vi "Configure_Run.vi"(8 "error in":errorcluster, 9 "Base Station":T1="BS1", 10 "Band":enum32{"GSM", "eNodeB", "gNodeB"}(ring)=enum."eNodeB", 11 "Input":T2={"Ref_Cluster"={"UE1"=refnum, "UE2"=refnum, "UE3"=refnum, "SelectNetwork1"=refnum, "SelectNetwork3"=refnum, "SelectNetwork2"=refnum, "Trace_Table1"=refnum, "UE - 1"=refnum, "UE - 2"=refnum, "UE - 3"=refnum, "UE - 4"=refnum, "Network-3"=refnum, "Status"=refnum, "Trace_Table2"=refnum, "UE4"=refnum, "Start"=refnum, "Reset"=refnum, "IP simulation"=refnum, "Network-1"=refnum, "Time Stamp"=refnum, "Network-2"=refnum, "IMS"=refnum, "GSM-Data"=refnum, "Configurations"=refnum, "Band"=refnum, "Sim Configurations"=refnum, "ECall"=refnum, "WWW"=refnum, "Cancel Configurations"=refnum, "GSM-PHY"=refnum, "GSM-CELL"=refnum, "GSM-GPRS"=refnum, "LTE-CELL"=refnum, "LTE-PHY"=refnum, "LTE-RRC"=refnum, "LTE-SDR"=refnum, "NR-RRC"=refnum, "NR-SDR"=refnum, "NR-PHY"=refnum, "NR-CELL"=refnum, "GSM-SDR"=refnum, "gNodeB-Data"=refnum, "eNodeB-Data"=refnum, "Select BS"=refnum, "Download"=refnum, "Upload"=refnum}, "Time Stamp"=timestamp(0 s since 1904-01-01), "Network-3"={"NW3-Thr-Down"=0.0, "NW3-Thr-Up"=0.0, "NW3-Fre-Down"=0.0, "NW3-Fre-Up"=0.0, "NW3-PwL-Down"=0.0, "NW3-PwL-Up"=0.0}, "Network-2"={"NW2-Thr-Down"=0.0, "NW2-Thr-Up"=0.0, "NW2-Fre-Down"=0.0, "NW2-Fre-Up"=0.0, "NW2-PwL-Down"=0.0, "NW2-PwL-Up"=0.0}, "Network-1"={"NW1-Thr-Down"=0.0, "NW1-Thr-Up"=0.0, "NW1-Fre-Down"=0.0, "NW1-Fre-Up"=0.0, "NW1-PwL-Down"=0.0, "NW1-PwL-Up"=0.0}, "UE - 4"={"UE4-Idle"=FALSE, "UE4-Origination"=FALSE, "UE4-Registration"=FALSE, "UE4-Pdu Connection"=FALSE, "UE4-Termination"=FALSE, "UE4-Detach"=FALSE}, "UE - 2"={"UE2-Idle"=FALSE, "UE2-Origination"=FALSE, "UE2-Registration"=FALSE, "UE2-Pdu Connection"=FALSE, "UE2-Termination"=FALSE, "UE2-Detach"=FALSE}, "UE - 1"={"UE1-Idle"=FALSE, "UE1-Origination"=FALSE, "UE1-Registration"=FALSE, "UE1-Pdu Connection"=FALSE, "UE1-Termination"=FALSE, "UE1-Detach"=FALSE}, "UE - 3"={"UE3-Idle"=FALSE, "UE3-Origination"=FALSE, "UE3-Registration"=FALSE, "UE3-Pdu Connection"=FALSE, "UE3-Termination"=FALSE, "UE3-Detach"=FALSE}, "IP simulation"=FALSE, "Start"=FALSE, "Reset"=FALSE, "Download"=FALSE, "Upload"=FALSE, "UE4"=FALSE, "UE3"=FALSE, "UE2"=FALSE, "UE1"=FALSE, "Trace_Table1"=0, "Status"="", "Trace_Table2"=0, "SelectNetwork1"={"Nw1-check"=FALSE, "NW-Combo"="GSM"}, "SelectNetwork2"={"Nw1-check"=FALSE, "NW-Combo"="GSM"}, "SelectNetwork3"={"Nw1-check"=FALSE, "NW-Combo"="GSM"}, "IMS"=FALSE, "WWW"=FALSE, "Sim Configuration"=FALSE, "Ecall"=FALSE, "Configurations"=enum."Configurations", "Band"=enum."GSM", "GSM-Data"=enum."SDR", "eNodeB-Data"=enum."RRC", "gNodeB-Data"=enum."SDR", "Cancel Configurations"=FALSE, "IP_UI"={"Add"=FALSE, "Close"=FALSE, "IP_UI"=[]}, "IMS_DATA"=[], "ECall DATA"=[], "Technology"="", "Sim Cluster in"={"Session_array"=[{"Add Bearer"=FALSE, "APN Name\n"="as", "AMBR Uplink(Gbps)\n"="as", "AMBR Downlink(Gbps)\n"="11111111111111111111111111111111", "Session name"="8baf473f2f8fd09487cccbd7097c6862", "Bearer_Array"=[], "Delete Session"=FALSE}], "SIM_U_Config"={"Add"=FALSE, "Close"=TRUE, "SIM_UI"=[], "Save"=FALSE}}, "Select BS"="", "Select Network 1"={"Network 1-2G"={"GSM-SDR"={"DL Reference Power"=-13, "Serail Name"="", "UL Reference Power"=-13, "Radio Device"="0"}, "GSM-GPRS"={"Priority Access THR"="6", "Acess Burst Type"="0", "Nack Countdown"="8", "BCCH/PDCH Measurement"="0", "Routing Area Code(RAC)"=128, "Network Control Order"="0", "t3168"="3", "t3192"="2", "Alpha"="10"}, "GSM-PHY"={"RACH Maximum Retransmission"="3", "RACH Transmission Slots"="1", "RACH Call Reestablishment"="1", "RACH Access Control Class"="1", "Block for Access Grant"="0", "Multiframe for Paging"="0", "Power Control Indicator"="0", "Radio Link Timeout"="850", "Cell Reselect Hysterisis"="0", "Attach/Detach Allowed"="0", "CCCH Combinations"="0", "t3212"=0, "DTX Indicator"="1", "Power Control Level"=0, "Minimum Received Signal Level"=0, "Half Rate Support"="0", "Add Reselect"="1"}, "GSM-CELL"={"SMS Enabled"="0", "Eutra Operating Bands"="3", "Power Offset Indicator"="", "Early Classmark Sending Control"="1", "Location Area Code"=0, "CALL Enabled"="1", "Loop Back Enabled"="0", "GPRS Enabled"="1", "SI Type 2 ter Indicator"="0", "ARFCN"=1, "Frequency Format ID"=1, "Mobile Country Code"=1, "Mobile Network Code"=1, "Cell Barred Access"="ONESIXTH", "Downlink Frequency"=-13, "Uplink Frequency"=1842}}, "Network 1-4G"={"LTE-SDR"={"Radio Device"="0", "DL Reference Power"=-13, "Serail Name"="", "UL Reference Power"=-13, "DL Antennas"="1", "UL Antennas"="1"}, "LTE-PHY"={"PBCH Repetition"="0", "PUCCH Delta Shift"="0", "PUCCH CQI Number of RB"="2", "PHICH Resource"="0", "SRS Enable"="0", "PCCH Paging Cycle"="1", "BCCH Modification Coefficient"="10", "PUSCH Alpha"="48", "PUSCH DMRS Enable"="4", "PHICH Duration"="10", "PUCCH HARQ Max Transmission"=-27, "PCCH Narrowband Count"="-108", "PUSCH Power Offset"=0, "PUCCH Power Offset"=0, "PDSCH Power Boost"="0", "PUCCH An Occassions"="1", "PUUCH CS Antenna Ports"="10", "PRACH Response Window Size"="MaxEye", "PRACH Contention Resolution Timer"="TM1", "PRACH Ramping Step Size"="2", "PDSCH Reference Power"=-27, "PRACH Root Sequence Index"=80, "PRACH Maximum Transmissions"="0", "PRACH Initial Received Target Power"="4", "PRACH Configuration Index"=98}, "LTE-CELL"={"Duplex Mode"="10", "Measurement Report"="1", "Eutra Operating Bands"="139", "Carrier Bandwidth"="10", "Physical Cell ID"=0, "Network Name"="one", "DL Frequency"=4, "UL Frequency"=25, "Transmission Mode"="TM1", "MNC Length"="77", "IMS Enabled"="1", "Tracking Area Code"=1, "Mobile Network Code"=1, "Mobile Country Code"=1}, "LTE-RRC"={"RLC Maximum Retransmision Threshold"="1", "RLC Timer Poll Retransmit"=0, "RLC Timer Reordering"=0, "RLC Timer Status Prohibit"=-96, "RLC Poll PDU"=13, "RLC Poll Byte"=1}}, "Network 1-5G"={"NR-SDR"={"DL Reference Power"=0, "Serail Name"="1", "UL Reference Power"=-13, "DL Antennas"="0", "UL Antennas"="0", "Radio Device"="1"}, "NR-PHY"={"PDSCH Reference Power"=-27, "SSB RSRP Threshold"=-109, "PRACH Contention Resolution Timer"=7, "Preamble Per SSB"=14, "Preamble Per SSB Format"=4, "UE Power Level Grant"=-90, "RA Response Window"="1", "Power Ramp Step Size"="2", "Preamble Root Sequence Index"="139", "Preamble Transmission Count"="10", "Preamble Received Power"=-96, "Zero Correlation Zone Configuration"=13, "Msg Frequency Division Multiplexing"="one", "PRACH Configuration Index"=98, "Preamble Timing Offset"=1, "Preamble Format"=0, "Resource Restriction Type"="0"}, "NR-CELL"={"Tracking Area Code"=1, "Mobile Country Code"=1, "Mobile Network Code"=1, "Operating Bands"="77", "Physical Cell ID"=0, "DL Offset to Carrier"=0, "Subcarrier Spacing"="1", "UL Offset to Carrier 2"=0, "Carrier Bandwidth"="10", "Transmission Mode"="TM1", "CSI-RS"="1", "SRS"="1", "Measurement Report"="1"}, "NR-RRC"={"Ciphering Algorithms for SRB"="0", "Integrity Algorithms for SRB"="0", "Ciphering Algorithms for DRB"="1", "Integrity Algorithms for DRB"="1"}}, "Technology-1"=""}, "Select Network 2"={"Network 2-2G"={"GSM-SDR"={"DL Reference Power"=-13, "Serail Name"="", "UL Reference Power"=-13, "Radio Device"="0"}, "GSM-GPRS"={"Priority Access THR"="6", "Acess Burst Type"="0", "Nack Countdown"="8", "BCCH/PDCH Measurement"="0", "Routing Area Code(RAC)"=128, "Network Control Order"="0", "t3168"="3", "t3192"="2", "Alpha"="10"}, "GSM-PHY"={"RACH Maximum Retransmission"="1", "RACH Transmission Slots"="14", "RACH Call Reestablishment"="1", "RACH Access Control Class"="0", "Block for Access Grant"="2", "Multiframe for Paging"="0", "Power Control Indicator"="0", "Radio Link Timeout"="15", "Cell Reselect Hysterisis"="3", "Attach/Detach Allowed"="1", "CCCH Combinations"="1", "t3212"=0, "DTX Indicator"="1", "Power Control Level"=0, "Minimum Received Signal Level"=0, "Half Rate Support"="0", "Add Reselect"="0"}, "GSM-CELL"={"SMS Enabled"="0", "Eutra Operating Bands"="850", "Power Offset Indicator"="0", "Early Classmark Sending Control"="0", "Location Area Code"=1, "CALL Enabled"="0", "Loop Back Enabled"="1", "GPRS Enabled"="0", "SI Type 2 ter Indicator"="1", "ARFCN"=0, "Frequency Format ID"=71, "Mobile Country Code"=1, "Mobile Network Code"=1, "Cell Barred Access"="0", "Downlink Frequency"=0, "Uplink Frequency"=900200000}}, "Network 2-4G"={"LTE-SDR"={"Radio Device"="0", "DL Reference Power"=-13, "Serail Name"="", "UL Reference Power"=-13, "DL Antennas"="1", "UL Antennas"="1"}, "LTE-PHY"={"PBCH Repetition"="0", "PUCCH Delta Shift"="1", "PUCCH CQI Number of RB"="0", "PHICH Resource"="ONESIXTH", "SRS Enable"="0", "PCCH Paging Cycle"="256", "BCCH Modification Coefficient"="2", "PUSCH Alpha"="1", "PUSCH DMRS Enable"="0", "PHICH Duration"="0", "PUCCH HARQ Max Transmission"=4, "PCCH Narrowband Count"="2", "PUSCH Power Offset"=-96, "PUCCH Power Offset"=-96, "PDSCH Power Boost"="0", "PUCCH An Occassions"="0", "PUUCH CS Antenna Ports"="1", "PRACH Response Window Size"="10", "PRACH Contention Resolution Timer"="48", "PRACH Ramping Step Size"="4", "PDSCH Reference Power"=-27, "PRACH Root Sequence Index"=0, "PRACH Maximum Transmissions"="10", "PRACH Initial Received Target Power"="-108", "PRACH Configuration Index"=0}, "LTE-CELL"={"Duplex Mode"="0", "Measurement Report"="1", "Eutra Operating Bands"="3", "Carrier Bandwidth"="10", "Physical Cell ID"=0, "Network Name"="MaxEye", "DL Frequency"=1842, "UL Frequency"=1747, "Transmission Mode"="TM1", "MNC Length"="2", "IMS Enabled"="0", "Tracking Area Code"=1, "Mobile Network Code"=1, "Mobile Country Code"=1}, "LTE-RRC"={"RLC Maximum Retransmision Threshold"="4", "RLC Timer Poll Retransmit"=80, "RLC Timer Reordering"=35, "RLC Timer Status Prohibit"=0, "RLC Poll PDU"=4, "RLC Poll Byte"=25}}, "Network 2-5G"={"NR-SDR"={"DL Reference Power"=-13, "Serail Name"="", "UL Reference Power"=-13, "DL Antennas"="1", "UL Antennas"="1", "Radio Device"="0"}, "NR-PHY"={"PDSCH Reference Power"=-27, "SSB RSRP Threshold"=-109, "PRACH Contention Resolution Timer"=7, "Preamble Per SSB"=14, "Preamble Per SSB Format"=4, "UE Power Level Grant"=-90, "RA Response Window"="10", "Power Ramp Step Size"="2", "Preamble Root Sequence Index"="139", "Preamble Transmission Count"="10", "Preamble Received Power"=-96, "Zero Correlation Zone Configuration"=13, "Msg Frequency Division Multiplexing"="one", "PRACH Configuration Index"=98, "Preamble Timing Offset"=1, "Preamble Format"=0, "Resource Restriction Type"="0"}, "NR-CELL"={"Tracking Area Code"=1, "Mobile Country Code"=1, "Mobile Network Code"=1, "Operating Bands"="77", "Physical Cell ID"=0, "DL Offset to Carrier"=0, "Subcarrier Spacing"="1", "UL Offset to Carrier 2"=0, "Carrier Bandwidth"="10", "Transmission Mode"="TM1", "CSI-RS"="1", "SRS"="1", "Measurement Report"="1"}, "NR-RRC"={"Ciphering Algorithms for SRB"="0", "Integrity Algorithms for SRB"="0", "Ciphering Algorithms for DRB"="1", "Integrity Algorithms for DRB"="1"}}, "Technology-2"=""}, "Select Network 3"={"Network 3-2G"={"GSM-SDR"={"DL Reference Power"=-13, "Serail Name"="", "UL Reference Power"=-13, "Radio Device"="0"}, "GSM-GPRS"={"Priority Access THR"="6", "Acess Burst Type"="0", "Nack Countdown"="8", "BCCH/PDCH Measurement"="0", "Routing Area Code(RAC)"=128, "Network Control Order"="0", "t3168"="3", "t3192"="2", "Alpha"="10"}, "GSM-PHY"={"RACH Maximum Retransmission"="1", "RACH Transmission Slots"="14", "RACH Call Reestablishment"="1", "RACH Access Control Class"="0", "Block for Access Grant"="2", "Multiframe for Paging"="0", "Power Control Indicator"="0", "Radio Link Timeout"="15", "Cell Reselect Hysterisis"="3", "Attach/Detach Allowed"="1", "CCCH Combinations"="1", "t3212"=0, "DTX Indicator"="1", "Power Control Level"=0, "Minimum Received Signal Level"=0, "Half Rate Support"="0", "Add Reselect"="0"}, "GSM-CELL"={"SMS Enabled"="0", "Eutra Operating Bands"="850", "Power Offset Indicator"="0", "Early Classmark Sending Control"="0", "Location Area Code"=1, "CALL Enabled"="0", "Loop Back Enabled"="1", "GPRS Enabled"="0", "SI Type 2 ter Indicator"="1", "ARFCN"=0, "Frequency Format ID"=71, "Mobile Country Code"=1, "Mobile Network Code"=1, "Cell Barred Access"="0", "Downlink Frequency"=0, "Uplink Frequency"=900200000}}, "Network 3-4G"={"LTE-SDR"={"Radio Device"="0", "DL Reference Power"=-13, "Serail Name"="", "UL Reference Power"=-13, "DL Antennas"="1", "UL Antennas"="1"}, "LTE-PHY"={"PBCH Repetition"="0", "PUCCH Delta Shift"="1", "PUCCH CQI Number of RB"="0", "PHICH Resource"="ONESIXTH", "SRS Enable"="0", "PCCH Paging Cycle"="256", "BCCH Modification Coefficient"="2", "PUSCH Alpha"="1", "PUSCH DMRS Enable"="0", "PHICH Duration"="0", "PUCCH HARQ Max Transmission"=4, "PCCH Narrowband Count"="2", "PUSCH Power Offset"=-96, "PUCCH Power Offset"=-96, "PDSCH Power Boost"="0", "PUCCH An Occassions"="0", "PUUCH CS Antenna Ports"="1", "PRACH Response Window Size"="10", "PRACH Contention Resolution Timer"="48", "PRACH Ramping Step Size"="4", "PDSCH Reference Power"=-27, "PRACH Root Sequence Index"=0, "PRACH Maximum Transmissions"="10", "PRACH Initial Received Target Power"="-108", "PRACH Configuration Index"=0}, "LTE-CELL"={"Duplex Mode"="0", "Measurement Report"="1", "Eutra Operating Bands"="3", "Carrier Bandwidth"="10", "Physical Cell ID"=0, "Network Name"="MaxEye", "DL Frequency"=1842, "UL Frequency"=1747, "Transmission Mode"="TM1", "MNC Length"="2", "IMS Enabled"="0", "Tracking Area Code"=1, "Mobile Network Code"=1, "Mobile Country Code"=1}, "LTE-RRC"={"RLC Maximum Retransmision Threshold"="4", "RLC Timer Poll Retransmit"=80, "RLC Timer Reordering"=35, "RLC Timer Status Prohibit"=0, "RLC Poll PDU"=4, "RLC Poll Byte"=25}}, "Network 3-5G"={"NR-SDR"={"DL Reference Power"=-13, "Serail Name"="", "UL Reference Power"=-13, "DL Antennas"="1", "UL Antennas"="1", "Radio Device"="0"}, "NR-PHY"={"PDSCH Reference Power"=-27, "SSB RSRP Threshold"=-109, "PRACH Contention Resolution Timer"=7, "Preamble Per SSB"=14, "Preamble Per SSB Format"=4, "UE Power Level Grant"=-90, "RA Response Window"="10", "Power Ramp Step Size"="2", "Preamble Root Sequence Index"="139", "Preamble Transmission Count"="10", "Preamble Received Power"=-96, "Zero Correlation Zone Configuration"=13, "Msg Frequency Division Multiplexing"="one", "PRACH Configuration Index"=98, "Preamble Timing Offset"=1, "Preamble Format"=0, "Resource Restriction Type"="0"}, "NR-CELL"={"Tracking Area Code"=1, "Mobile Country Code"=1, "Mobile Network Code"=1, "Operating Bands"="77", "Physical Cell ID"=0, "DL Offset to Carrier"=0, "Subcarrier Spacing"="1", "UL Offset to Carrier 2"=0, "Carrier Bandwidth"="10", "Transmission Mode"="TM1", "CSI-RS"="1", "SRS"="1", "Measurement Report"="1"}, "NR-RRC"={"Ciphering Algorithms for SRB"="0", "Integrity Algorithms for SRB"="0", "Ciphering Algorithms for DRB"="1", "Integrity Algorithms for DRB"="1"}}, "Technology-3"=""}, "Current Technology"="", "Current Network"=""} {"Time Stamp" format="%<%H:%M:%S>T"}) -> (0 "error out":errorcluster)   [LabVIEW 2021]
uses:
  Controls/ATE_BSE_Controls_ref.ctl
  Controls/ATE_BSE_ref_type_Def.ctl
  IP Simulation/Controls/IP_Cellular Tech Type def.ctl
  IP Simulation/Controls/IP_Network_Type def.ctl
  IP Simulation/Controls/IP_Type-Tydedef.ctl
  Save File/Sim_Confi.ctl
  APIs/Controls/Base_Station_Emulator.ctl
  APIs/Controls/Cellular_Technology.ctl
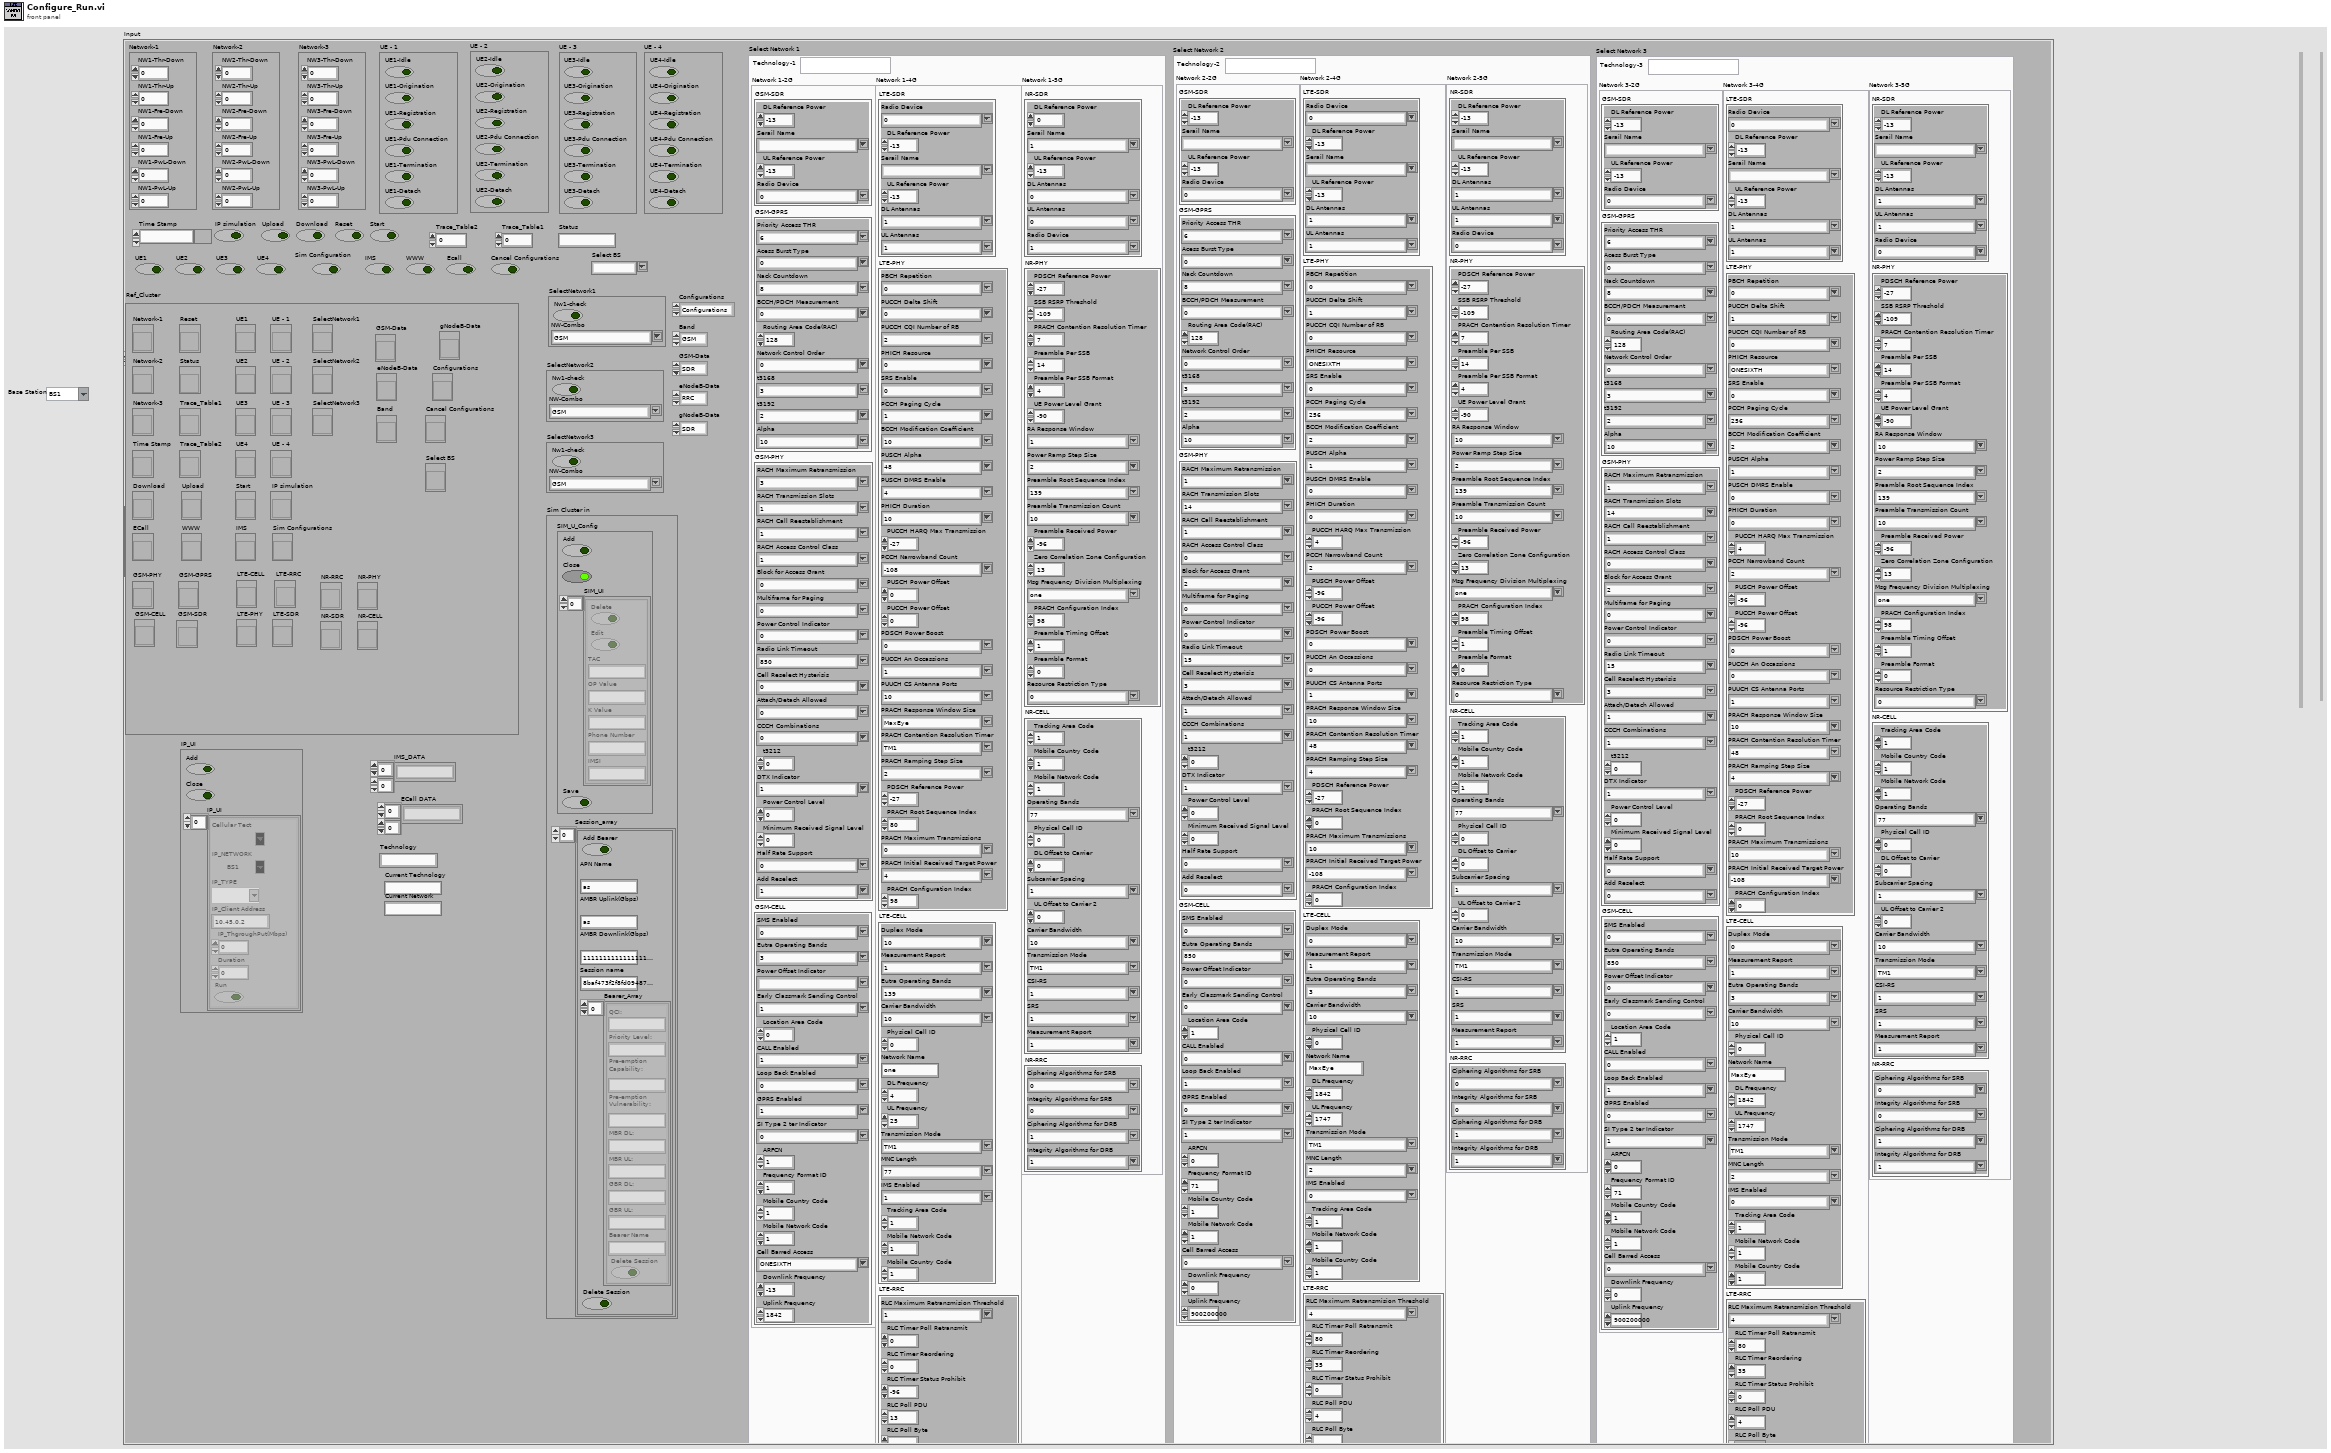
[diagram p1: front panel]
types:
  T1 = typedef "Base_Station_Emulator.ctl" = string
  T2 = typedef "ATE_BSE_Controls_ref.ctl" = cluster{"Ref_Cluster":T3, "Time Stamp":timestamp, "Network-3":cluster{"NW3-Thr-Down":dbl, "NW3-Thr-Up":dbl, "NW3-Fre-Down":dbl, "NW3-Fre-Up":dbl, "NW3-PwL-Down":dbl, "NW3-PwL-Up":dbl}, "Network-2":cluster{"NW2-Thr-Down":dbl, "NW2-Thr-Up":dbl, "NW2-Fre-Down":dbl, "NW2-Fre-Up":dbl, "NW2-PwL-Down":dbl, "NW2-PwL-Up":dbl}, "Network-1":cluster{"NW1-Thr-Down":dbl, "NW1-Thr-Up":dbl, "NW1-Fre-Down":dbl, "NW1-Fre-Up":dbl, "NW1-PwL-Down":dbl, "NW1-PwL-Up":dbl}, "UE - 4":cluster{"UE4-Idle":bool, "UE4-Origination":bool, "UE4-Registration":bool, "UE4-Pdu Connection":bool, "UE4-Termination":bool, "UE4-Detach":bool}, "UE - 2":cluster{"UE2-Idle":bool, "UE2-Origination":bool, "UE2-Registration":bool, "UE2-Pdu Connection":bool, "UE2-Termination":bool, "UE2-Detach":bool}, "UE - 1":cluster{"UE1-Idle":bool, "UE1-Origination":bool, "UE1-Registration":bool, "UE1-Pdu Connection":bool, "UE1-Termination":bool, "UE1-Detach":bool}, "UE - 3":cluster{"UE3-Idle":bool, "UE3-Origination":bool, "UE3-Registration":bool, "UE3-Pdu Connection":bool, "UE3-Termination":bool, "UE3-Detach":bool}, "IP simulation":bool, "Start":bool, "Reset":bool, "Download":bool, "Upload":bool, "UE4":bool, "UE3":bool, "UE2":bool, "UE1":bool, "Trace_Table1":i32, "Status":string, "Trace_Table2":i32, "SelectNetwork1":cluster{"Nw1-check":bool, "NW-Combo":string}, "SelectNetwork2":cluster{"Nw1-check":bool, "NW-Combo":string}, "SelectNetwork3":cluster{"Nw1-check":bool, "NW-Combo":string}, "IMS":bool, "WWW":bool, "Sim Configuration":bool, "Ecall":bool, "Configurations":enum32{"Configurations", "Main"}, "Band":enum32{"GSM", "gNodeB", "eNodeB"}, "GSM-Data":enum32{"SDR", "CELL", "PHY", "GPRS"}, "eNodeB-Data":enum32{"SDR", "CELL", "PHY", "RRC"}, "gNodeB-Data":enum32{"SDR", "CELL", "PHY", "RRC"}, "Cancel Configurations":bool, "IP_UI":cluster{"Add":bool, "Close":bool, "IP_UI":cluster{"Cellular Tect":T4, "IP_NETWORK":T5, "IP_TYPE":T6, "IP_Client Address":string, "IP_ThgroughPut(Mbps)":i32, "Duration":i32, "Run":bool}[]}, "IMS_DATA":string[][], "ECall DATA":string[][], "Technology":string, "Sim Cluster in":T7, "Select BS":string, "Select Network 1":cluster{"Network 1-2G":cluster{"GSM-SDR":cluster{"DL Reference Power":i32, "Serail Name":string, "UL Reference Power":i32, "Radio Device":string}, "GSM-GPRS":cluster{"Priority Access THR":string, "Acess Burst Type":string, "Nack Countdown":string, "BCCH/PDCH Measurement":string, "Routing Area Code(RAC)":i32, "Network Control Order":string, "t3168":string, "t3192":string, "Alpha":string}, "GSM-PHY":cluster{"RACH Maximum Retransmission":string, "RACH Transmission Slots":string, "RACH Call Reestablishment":string, "RACH Access Control Class":string, "Block for Access Grant":string, "Multiframe for Paging":string, "Power Control Indicator":string, "Radio Link Timeout":string, "Cell Reselect Hysterisis":string, "Attach/Detach Allowed":string, "CCCH Combinations":string, "t3212":i64, "DTX Indicator":string, "Power Control Level":i64, "Minimum Received Signal Level":i64, "Half Rate Support":string, "Add Reselect":string}, "GSM-CELL":cluster{"SMS Enabled":string, "Eutra Operating Bands":string, "Power Offset Indicator":string, "Early Classmark Sending Control":string, "Location Area Code":i32, "CALL Enabled":string, "Loop Back Enabled":string, "GPRS Enabled":string, "SI Type 2 ter Indicator":string, "ARFCN":i64, "Frequency Format ID":i64, "Mobile Country Code":i64, "Mobile Network Code":i64, "Cell Barred Access":string, "Downlink Frequency":i32, "Uplink Frequency":i32}}, "Network 1-4G":cluster{"LTE-SDR":cluster{"Radio Device":string, "DL Reference Power":i32, "Serail Name":string, "UL Reference Power":i32, "DL Antennas":string, "UL Antennas":string}, "LTE-PHY":cluster{"PBCH Repetition":string, "PUCCH Delta Shift":string, "PUCCH CQI Number of RB":string, "PHICH Resource":string, "SRS Enable":string, "PCCH Paging Cycle":string, "BCCH Modification Coefficient":string, "PUSCH Alpha":string, "PUSCH DMRS Enable":string, "PHICH Duration":string, "PUCCH HARQ Max Transmission":i64, "PCCH Narrowband Count":string, "PUSCH Power Offset":i64, "PUCCH Power Offset":i64, "PDSCH Power Boost":string, "PUCCH An Occassions":string, "PUUCH CS Antenna Ports":string, "PRACH Response Window Size":string, "PRACH Contention Resolution Timer":string, "PRACH Ramping Step Size":string, "PDSCH Reference Power":i64, "PRACH Root Sequence Index":i64, "PRACH Maximum Transmissions":string, "PRACH Initial Received Target Power":string, "PRACH Configuration Index":i64}, "LTE-CELL":cluster{"Duplex Mode":string, "Measurement Report":string, "Eutra Operating Bands":string, "Carrier Bandwidth":string, "Physical Cell ID":i64, "Network Name":string, "DL Frequency":i32, "UL Frequency":i32, "Transmission Mode":string, "MNC Length":string, "IMS Enabled":string, "Tracking Area Code":i32, "Mobile Network Code":i32, "Mobile Country Code":i32}, "LTE-RRC":cluster{"RLC Maximum Retransmision Threshold":string, "RLC Timer Poll Retransmit":i32, "RLC Timer Reordering":i32, "RLC Timer Status Prohibit":i32, "RLC Poll PDU":i32, "RLC Poll Byte":i32}}, "Network 1-5G":cluster{"NR-SDR":cluster{"DL Reference Power":i32, "Serail Name":string, "UL Reference Power":i32, "DL Antennas":string, "UL Antennas":string, "Radio Device":string}, "NR-PHY":cluster{"PDSCH Reference Power":i64, "SSB RSRP Threshold":i64, "PRACH Contention Resolution Timer":i64, "Preamble Per SSB":i64, "Preamble Per SSB Format":i64, "UE Power Level Grant":i64, "RA Response Window":string, "Power Ramp Step Size":string, "Preamble Root Sequence Index":string, "Preamble Transmission Count":string, "Preamble Received Power":i64, "Zero Correlation Zone Configuration":i64, "Msg Frequency Division Multiplexing":string, "PRACH Configuration Index":i64, "Preamble Timing Offset":i64, "Preamble Format":i64, "Resource Restriction Type":string}, "NR-CELL":cluster{"Tracking Area Code":i64, "Mobile Country Code":i64, "Mobile Network Code":i64, "Operating Bands":string, "Physical Cell ID":i64, "DL Offset to Carrier":i32, "Subcarrier Spacing":string, "UL Offset to Carrier 2":i32, "Carrier Bandwidth":string, "Transmission Mode":string, "CSI-RS":string, "SRS":string, "Measurement Report":string}, "NR-RRC":cluster{"Ciphering Algorithms for SRB":string, "Integrity Algorithms for SRB":string, "Ciphering Algorithms for DRB":string, "Integrity Algorithms for DRB":string}}, "Technology-1":string}, "Select Network 2":cluster{"Network 2-2G":cluster{"GSM-SDR":cluster{"DL Reference Power":i32, "Serail Name":string, "UL Reference Power":i32, "Radio Device":string}, "GSM-GPRS":cluster{"Priority Access THR":string, "Acess Burst Type":string, "Nack Countdown":string, "BCCH/PDCH Measurement":string, "Routing Area Code(RAC)":i32, "Network Control Order":string, "t3168":string, "t3192":string, "Alpha":string}, "GSM-PHY":cluster{"RACH Maximum Retransmission":string, "RACH Transmission Slots":string, "RACH Call Reestablishment":string, "RACH Access Control Class":string, "Block for Access Grant":string, "Multiframe for Paging":string, "Power Control Indicator":string, "Radio Link Timeout":string, "Cell Reselect Hysterisis":string, "Attach/Detach Allowed":string, "CCCH Combinations":string, "t3212":i64, "DTX Indicator":string, "Power Control Level":i64, "Minimum Received Signal Level":i64, "Half Rate Support":string, "Add Reselect":string}, "GSM-CELL":cluster{"SMS Enabled":string, "Eutra Operating Bands":string, "Power Offset Indicator":string, "Early Classmark Sending Control":string, "Location Area Code":i32, "CALL Enabled":string, "Loop Back Enabled":string, "GPRS Enabled":string, "SI Type 2 ter Indicator":string, "ARFCN":i64, "Frequency Format ID":i64, "Mobile Country Code":i64, "Mobile Network Code":i64, "Cell Barred Access":string, "Downlink Frequency":i32, "Uplink Frequency":i32}}, "Network 2-4G":cluster{"LTE-SDR":cluster{"Radio Device":string, "DL Reference Power":i32, "Serail Name":string, "UL Reference Power":i32, "DL Antennas":string, "UL Antennas":string}, "LTE-PHY":cluster{"PBCH Repetition":string, "PUCCH Delta Shift":string, "PUCCH CQI Number of RB":string, "PHICH Resource":string, "SRS Enable":string, "PCCH Paging Cycle":string, "BCCH Modification Coefficient":string, "PUSCH Alpha":string, "PUSCH DMRS Enable":string, "PHICH Duration":string, "PUCCH HARQ Max Transmission":i64, "PCCH Narrowband Count":string, "PUSCH Power Offset":i64, "PUCCH Power Offset":i64, "PDSCH Power Boost":string, "PUCCH An Occassions":string, "PUUCH CS Antenna Ports":string, "PRACH Response Window Size":string, "PRACH Contention Resolution Timer":string, "PRACH Ramping Step Size":string, "PDSCH Reference Power":i64, "PRACH Root Sequence Index":i64, "PRACH Maximum Transmissions":string, "PRACH Initial Received Target Power":string, "PRACH Configuration Index":i64}, "LTE-CELL":cluster{"Duplex Mode":string, "Measurement Report":string, "Eutra Operating Bands":string, "Carrier Bandwidth":string, "Physical Cell ID":i64, "Network Name":string, "DL Frequency":i32, "UL Frequency":i32, "Transmission Mode":string, "MNC Length":string, "IMS Enabled":string, "Tracking Area Code":i32, "Mobile Network Code":i32, "Mobile Country Code":i32}, "LTE-RRC":cluster{"RLC Maximum Retransmision Threshold":string, "RLC Timer Poll Retransmit":i32, "RLC Timer Reordering":i32, "RLC Timer Status Prohibit":i32, "RLC Poll PDU":i32, "RLC Poll Byte":i32}}, "Network 2-5G":cluster{"NR-SDR":cluster{"DL Reference Power":i32, "Serail Name":string, "UL Reference Power":i32, "DL Antennas":string, "UL Antennas":string, "Radio Device":string}, "NR-PHY":cluster{"PDSCH Reference Power":i64, "SSB RSRP Threshold":i64, "PRACH Contention Resolution Timer":i64, "Preamble Per SSB":i64, "Preamble Per SSB Format":i64, "UE Power Level Grant":i64, "RA Response Window":string, "Power Ramp Step Size":string, "Preamble Root Sequence Index":string, "Preamble Transmission Count":string, "Preamble Received Power":i64, "Zero Correlation Zone Configuration":i64, "Msg Frequency Division Multiplexing":string, "PRACH Configuration Index":i64, "Preamble Timing Offset":i64, "Preamble Format":i64, "Resource Restriction Type":string}, "NR-CELL":cluster{"Tracking Area Code":i64, "Mobile Country Code":i64, "Mobile Network Code":i64, "Operating Bands":string, "Physical Cell ID":i64, "DL Offset to Carrier":i32, "Subcarrier Spacing":string, "UL Offset to Carrier 2":i32, "Carrier Bandwidth":string, "Transmission Mode":string, "CSI-RS":string, "SRS":string, "Measurement Report":string}, "NR-RRC":cluster{"Ciphering Algorithms for SRB":string, "Integrity Algorithms for SRB":string, "Ciphering Algorithms for DRB":string, "Integrity Algorithms for DRB":string}}, "Technology-2":string}, "Select Network 3":cluster{"Network 3-2G":cluster{"GSM-SDR":cluster{"DL Reference Power":i32, "Serail Name":string, "UL Reference Power":i32, "Radio Device":string}, "GSM-GPRS":cluster{"Priority Access THR":string, "Acess Burst Type":string, "Nack Countdown":string, "BCCH/PDCH Measurement":string, "Routing Area Code(RAC)":i32, "Network Control Order":string, "t3168":string, "t3192":string, "Alpha":string}, "GSM-PHY":cluster{"RACH Maximum Retransmission":string, "RACH Transmission Slots":string, "RACH Call Reestablishment":string, "RACH Access Control Class":string, "Block for Access Grant":string, "Multiframe for Paging":string, "Power Control Indicator":string, "Radio Link Timeout":string, "Cell Reselect Hysterisis":string, "Attach/Detach Allowed":string, "CCCH Combinations":string, "t3212":i64, "DTX Indicator":string, "Power Control Level":i64, "Minimum Received Signal Level":i64, "Half Rate Support":string, "Add Reselect":string}, "GSM-CELL":cluster{"SMS Enabled":string, "Eutra Operating Bands":string, "Power Offset Indicator":string, "Early Classmark Sending Control":string, "Location Area Code":i32, "CALL Enabled":string, "Loop Back Enabled":string, "GPRS Enabled":string, "SI Type 2 ter Indicator":string, "ARFCN":i64, "Frequency Format ID":i64, "Mobile Country Code":i64, "Mobile Network Code":i64, "Cell Barred Access":string, "Downlink Frequency":i32, "Uplink Frequency":i32}}, "Network 3-4G":cluster{"LTE-SDR":cluster{"Radio Device":string, "DL Reference Power":i32, "Serail Name":string, "UL Reference Power":i32, "DL Antennas":string, "UL Antennas":string}, "LTE-PHY":cluster{"PBCH Repetition":string, "PUCCH Delta Shift":string, "PUCCH CQI Number of RB":string, "PHICH Resource":string, "SRS Enable":string, "PCCH Paging Cycle":string, "BCCH Modification Coefficient":string, "PUSCH Alpha":string, "PUSCH DMRS Enable":string, "PHICH Duration":string, "PUCCH HARQ Max Transmission":i64, "PCCH Narrowband Count":string, "PUSCH Power Offset":i64, "PUCCH Power Offset":i64, "PDSCH Power Boost":string, "PUCCH An Occassions":string, "PUUCH CS Antenna Ports":string, "PRACH Response Window Size":string, "PRACH Contention Resolution Timer":string, "PRACH Ramping Step Size":string, "PDSCH Reference Power":i64, "PRACH Root Sequence Index":i64, "PRACH Maximum Transmissions":string, "PRACH Initial Received Target Power":string, "PRACH Configuration Index":i64}, "LTE-CELL":cluster{"Duplex Mode":string, "Measurement Report":string, "Eutra Operating Bands":string, "Carrier Bandwidth":string, "Physical Cell ID":i64, "Network Name":string, "DL Frequency":i32, "UL Frequency":i32, "Transmission Mode":string, "MNC Length":string, "IMS Enabled":string, "Tracking Area Code":i32, "Mobile Network Code":i32, "Mobile Country Code":i32}, "LTE-RRC":cluster{"RLC Maximum Retransmision Threshold":string, "RLC Timer Poll Retransmit":i32, "RLC Timer Reordering":i32, "RLC Timer Status Prohibit":i32, "RLC Poll PDU":i32, "RLC Poll Byte":i32}}, "Network 3-5G":cluster{"NR-SDR":cluster{"DL Reference Power":i32, "Serail Name":string, "UL Reference Power":i32, "DL Antennas":string, "UL Antennas":string, "Radio Device":string}, "NR-PHY":cluster{"PDSCH Reference Power":i64, "SSB RSRP Threshold":i64, "PRACH Contention Resolution Timer":i64, "Preamble Per SSB":i64, "Preamble Per SSB Format":i64, "UE Power Level Grant":i64, "RA Response Window":string, "Power Ramp Step Size":string, "Preamble Root Sequence Index":string, "Preamble Transmission Count":string, "Preamble Received Power":i64, "Zero Correlation Zone Configuration":i64, "Msg Frequency Division Multiplexing":string, "PRACH Configuration Index":i64, "Preamble Timing Offset":i64, "Preamble Format":i64, "Resource Restriction Type":string}, "NR-CELL":cluster{"Tracking Area Code":i64, "Mobile Country Code":i64, "Mobile Network Code":i64, "Operating Bands":string, "Physical Cell ID":i64, "DL Offset to Carrier":i32, "Subcarrier Spacing":string, "UL Offset to Carrier 2":i32, "Carrier Bandwidth":string, "Transmission Mode":string, "CSI-RS":string, "SRS":string, "Measurement Report":string}, "NR-RRC":cluster{"Ciphering Algorithms for SRB":string, "Integrity Algorithms for SRB":string, "Ciphering Algorithms for DRB":string, "Integrity Algorithms for DRB":string}}, "Technology-3":string}, "Current Technology":string, "Current Network":string}
  T3 = typedef "ATE_BSE_ref_type_Def.ctl" = cluster{"UE1":refnum<vi>, "UE2":refnum<vi>, "UE3":refnum<vi>, "SelectNetwork1":refnum<vi>, "SelectNetwork3":refnum<vi>, "SelectNetwork2":refnum<vi>, "Trace_Table1":refnum<vi>, "UE - 1":refnum<vi>, "UE - 2":refnum<vi>, "UE - 3":refnum<vi>, "UE - 4":refnum<vi>, "Network-3":refnum<vi>, "Status":refnum<vi>, "Trace_Table2":refnum<vi>, "UE4":refnum<vi>, "Start":refnum<vi>, "Reset":refnum<vi>, "IP simulation":refnum<vi>, "Network-1":refnum<vi>, "Time Stamp":refnum<vi>, "Network-2":refnum<vi>, "IMS":refnum<vi>, "GSM-Data":refnum<vi>, "Configurations":refnum<vi>, "Band":refnum<vi>, "Sim Configurations":refnum<vi>, "ECall":refnum<vi>, "WWW":refnum<vi>, "Cancel Configurations":refnum<vi>, "GSM-PHY":refnum<vi>, "GSM-CELL":refnum<vi>, "GSM-GPRS":refnum<vi>, "LTE-CELL":refnum<vi>, "LTE-PHY":refnum<vi>, "LTE-RRC":refnum<vi>, "LTE-SDR":refnum<vi>, "NR-RRC":refnum<vi>, "NR-SDR":refnum<vi>, "NR-PHY":refnum<vi>, "NR-CELL":refnum<vi>, "GSM-SDR":refnum<vi>, "gNodeB-Data":refnum<vi>, "eNodeB-Data":refnum<vi>, "Select BS":refnum<vi>, "Download":refnum<vi>, "Upload":refnum<vi>}
  T4 = typedef "IP_Cellular Tech Type def.ctl" = string
  T5 = typedef "IP_Network_Type def.ctl" = string
  T6 = typedef "IP_Type-Tydedef.ctl" = string
  T7 = typedef "Sim_Confi.ctl" = cluster{"Session_array":cluster{"Add Bearer":bool, "APN Name\n":string, "AMBR Uplink(Gbps)\n":string, "AMBR Downlink(Gbps)\n":string, "Session name":string, "Bearer_Array":cluster{"QCI:":string, "Priority Level:":string, "Pre-emption\nCapability:":string, "Pre-emption\nVulnerability:":string, "MBR DL:":string, "MBR UL:":string, "GBR DL:":string, "GBR UL:":string, "Bearer Name":string, "Delete Session":bool}[], "Delete Session":bool}[], "SIM_U_Config":cluster{"Add":bool, "Close":bool, "SIM_UI":cluster{"Delete":bool, "Edit":bool, "TAC":string, "OP Value":string, "K Value":string, "Phone Number":string, "IMSI":string}[], "Save":bool}}
  T8 = typedef "Cellular_Technology.ctl" = string
  T9 = enum16{"Radio Device", "Serial name", "dl power", "ul ref power"}[]
  T10 = cluster{"DL Reference Power":i32, "Serial Name":string, "UL Reference Power":i32, "Radio Device":string}
  T11 = enum16{"Ul Frequency", "Dl Frequency", "Eutra Operating Bands", "arfcn", "call enables", "cell barred access", "early classmark sending", "fre format", "gprs enabled", "location aea code", "loop back enabled", "mcc", "mnc", "power offset", "si type", "sms enabled"}[]
  T12 = cluster{"SMS Enabled":string, "Eutra Operating Bands":string, "Power Offset Indicator":string, "Early Classmark Sending Control":string, "Location Area Code":i32, "CALL Enabled":string, "Loop Back Enabled":string, "GPRS Enabled":string, "SI Type 2 ter Indicator":string, "ARFCN":i64, "Frequency Format ID":i64, "Mobile Country Code":i64, "Mobile Network Code":i64, "Cell Barred Access":string, "Downlink Frequency":i32, "Uplink Frequency":i32}
  T13 = enum16{"ccch", "add reselect", "attach detach", "block for acs", "cell reselect", "dtx", "hal rate", "min received sig", "multiframe forpg", "pow con indi", "pow contro level", "Rach access control access", "rach call", "RAch maxi retranmission", "rach transmission slots", "radio link timout", "t3212"}[]
  T14 = cluster{"RACH Maximum Retransmission":string, "RACH Transmission Slots":string, "RACH Call Reestablishment":string, "RACH Access Control Class":string, "Block for Access Grant":string, "Multiframe for Paging":string, "Power Control Indicator":string, "Radio Link Timeout":string, "Cell Reselect Hysterisis":string, "Attach/Detach Allowed":string, "CCCH Combinations":string, "t3212":i64, "DTX Indicator":string, "Power Control Level":i64, "Minimum Received Signal Level":i64, "Half Rate Support":string, "Add Reselect":string}
  T15 = enum16{"bcch pdch", "gprs parameter alpha", "access burst", "nack countdown", "network control", "priority access", "rac", "t3168", "t3192"}[]
  T16 = cluster{"Priority Access THR":string, "Acess Burst Type":string, "Nack Countdown":string, "BCCH/PDCH Measurement":string, "Routing Area Code(RAC)":i32, "Network Control Order":string, "t3168":string, "t3192":string, "Alpha":string}
  T17 = enum16{"Radio Device", "Serial name", "dl power", "ul ref power", "Ul Antennas", "Dl Antennas"}[]
  T18 = cluster{"Radio Device":string, "DL Reference Power":i32, "Serail Name":string, "UL Reference Power":i32, "DL Antennas":string, "UL Antennas":string}
  T19 = enum16{"Carrier BW", "DL Frequency", "Duplex Mode", "Eutra operating band", "Measurement report", "MNC length", "MCC", "MNC", "network name", "Physical Cell ID", "Tracking area code", "Transmission Mode", "IMS Enable", "UL frequency"}[]
  T20 = cluster{"Duplex Mode":string, "Measurement Report":string, "Eutra Operating Bands":string, "Carrier Bandwidth":string, "Physical Cell ID":i64, "Network Name":string, "DL Frequency":i32, "UL Frequency":i32, "Transmission Mode":string, "MNC Length":string, "IMS Enabled":string, "Tracking Area Code":i32, "Mobile Network Code":i32, "Mobile Country Code":i32}
  T21 = enum16{"BCCH modi Coeff", "pbch Repetition", "pcch Narrowband", "pcch pg cycle", "pdsch power boost", "pdsch Ref power", "phich duration", "phish resource", "prach config index", "prach contention resolution", "prach initial received target", "prach maximum transmission", "prach ramping step size", "prach response window", "prach root sequence", "pussh an occassions", "pucch cqi num of RB", "pucch cs antenna", "pucch delta shift", "pucch harq max", "pucch power offset", "pusch alpha", "pusch dmrs enable", "pusch power offset", "srs enable"}[]
  T22 = cluster{"PBCH Repetition":string, "PUCCH Delta Shift":string, "PUCCH CQI Number of RB":string, "PHICH Resource":string, "SRS Enable":string, "PCCH Paging Cycle":string, "BCCH Modification Coefficient":string, "PUSCH Alpha":string, "PUSCH DMRS Enable":string, "PHICH Duration":string, "PUCCH HARQ Max Transmission":i64, "PCCH Narrowband Count":string, "PUSCH Power Offset":i64, "PUCCH Power Offset":i64, "PDSCH Power Boost":string, "PUCCH An Occassions":string, "PUUCH CS Antenna Ports":string, "PRACH Response Window Size":string, "PRACH Contention Resolution Timer":string, "PRACH Ramping Step Size":string, "PDSCH Reference Power":i64, "PRACH Root Sequence Index":i64, "PRACH Maximum Transmissions":string, "PRACH Initial Received Target Power":string, "PRACH Configuration Index":i64}
  T23 = enum16{"rlc maxi retransmission", "rlc poll byte", "rlc poll pdu", "rlc timer poll retransmit", "rlc timer reordering", "rlc timer status prohibit"}[]
  T24 = cluster{"RLC Maximum Retransmision Threshold":string, "RLC Timer Poll Retransmit":i32, "RLC Timer Reordering":i32, "RLC Timer Status Prohibit":i32, "RLC Poll PDU":i32, "RLC Poll Byte":i32}
  T25 = cluster{"DL Reference Power":i32, "Serail Name":string, "UL Reference Power":i32, "DL Antennas":string, "UL Antennas":string, "Radio Device":string}
  T26 = enum16{"Carrier Bandwidth", "CSI RS", "DL offset to Carrier", "Measurement Report", "Mobile Country code", "Mobile Network Code", "Operating Band", "Physical Cell ID", "SRS", "Subcarrier Spacing", "Tracking Area code", "Transmission Mode", "UL Offset to arrier"}[]
  T27 = cluster{"Tracking Area Code":i64, "Mobile Country Code":i64, "Mobile Network Code":i64, "Operating Bands":string, "Physical Cell ID":i64, "DL Offset to Carrier":i32, "Subcarrier Spacing":string, "UL Offset to Carrier 2":i32, "Carrier Bandwidth":string, "Transmission Mode":string, "CSI-RS":string, "SRS":string, "Measurement Report":string}
  T28 = enum16{"PDSCH Reference Power", "SSB RSRP Threshold", "PRACH Contention Resolution Timer", "Preamble Per SSB", "Preamble Per SSB Format", "UE Power Level Count", "RA Response Window", "Power Ramp Step Size", "Preamble Root Sequence Index", "Preamble Transmission  Count", "Preamble Received Power", "Zero Correlation Zone Configuration", "Msg Frequncy Division Multiplexing", "PRACH Configuration Index", "Preamble Timing Offset", "Preamble Format", "Resource Restriction Type"}[]
  T29 = cluster{"PDSCH Reference Power":i64, "SSB RSRP Threshold":i64, "PRACH Contention Resolution Timer":i64, "Preamble Per SSB":i64, "Preamble Per SSB Format":i64, "UE Power Level Grant":i64, "RA Response Window":string, "Power Ramp Step Size":string, "Preamble Root Sequence Index":string, "Preamble Transmission Count":string, "Preamble Received Power":i64, "Zero Correlation Zone Configuration":i64, "Msg Frequency Division Multiplexing":string, "PRACH Configuration Index":i64, "Preamble Timing Offset":i64, "Preamble Format":i64, "Resource Restriction Type":string}
  T30 = enum16{"Ciphering Algorithms for SRB", "Integrity Algorithms for SRB", "Ciphering Algorithms for DRB", "Integrity Algorithms for DRB"}[]
  T31 = cluster{"Ciphering Algorithms for SRB":string, "Integrity Algorithms for SRB":string, "Ciphering Algorithms for DRB":string, "Integrity Algorithms for DRB":string}
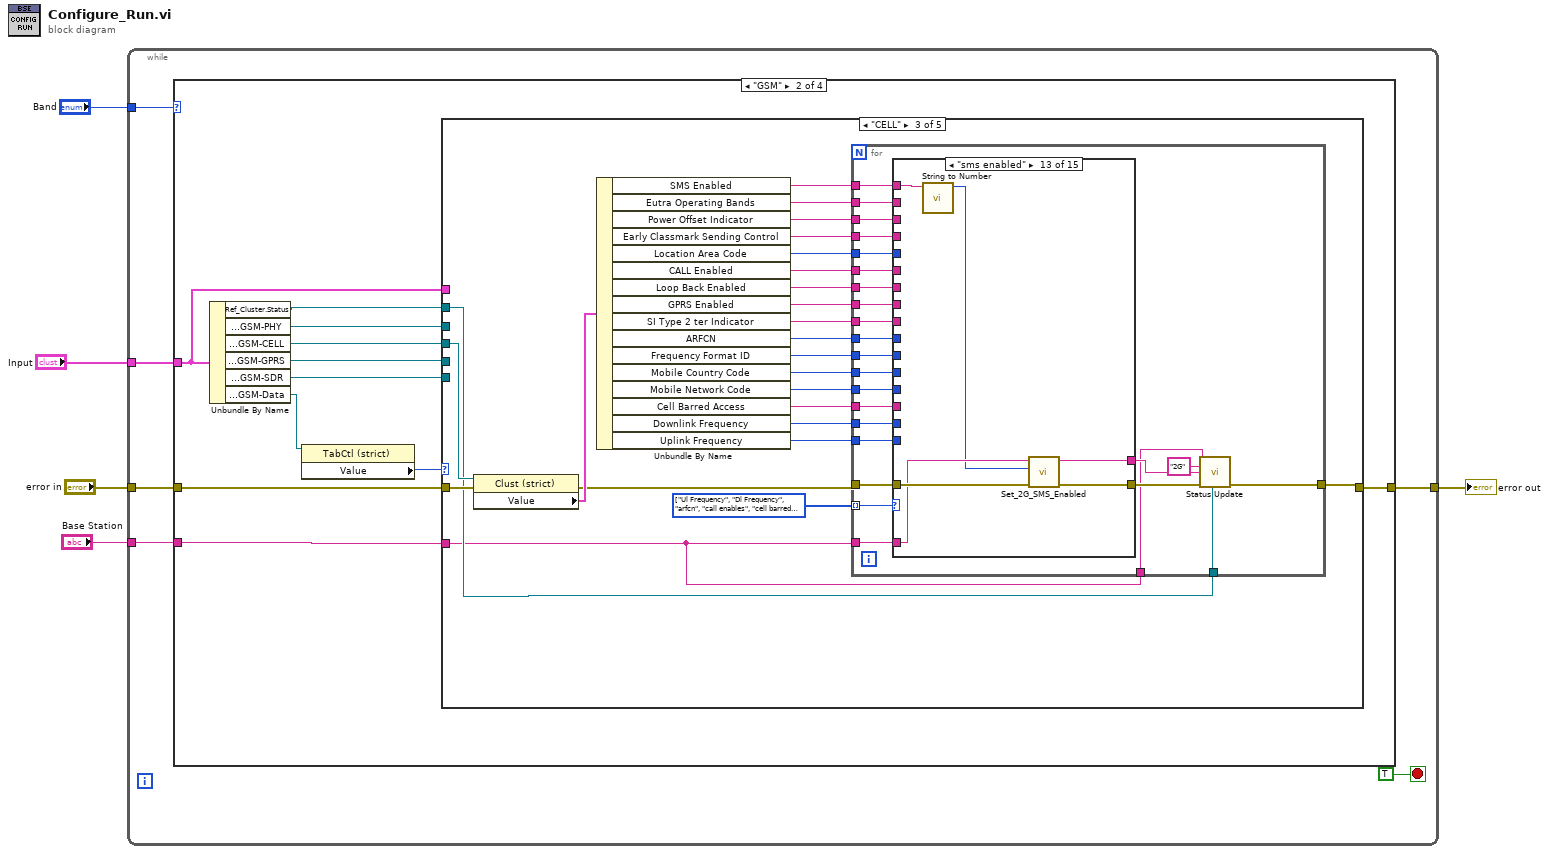
[diagram p0: block diagram]
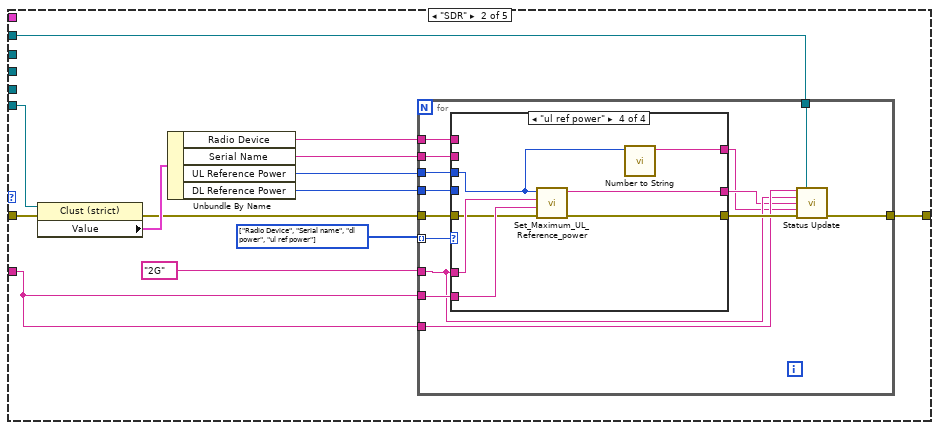
[diagram p4: hidden frame]
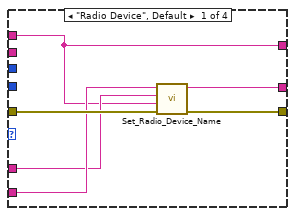
[diagram p5: hidden frame]
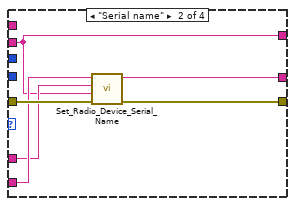
[diagram p6: hidden frame]
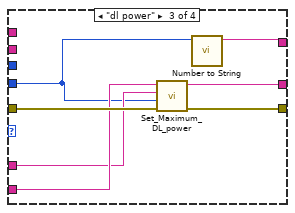
[diagram p7: hidden frame]
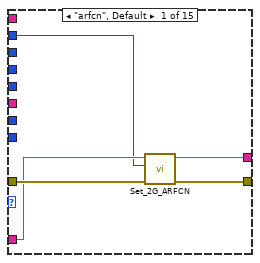
[diagram p8: hidden frame]
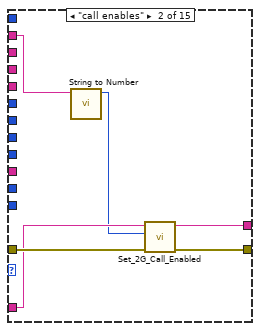
[diagram p9: hidden frame]
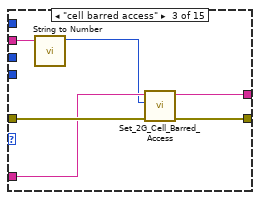
[diagram p10: hidden frame]
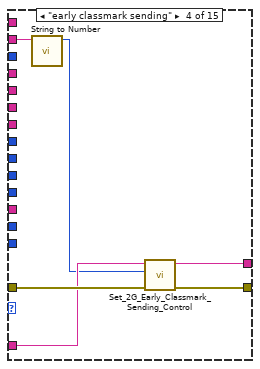
[diagram p11: hidden frame]
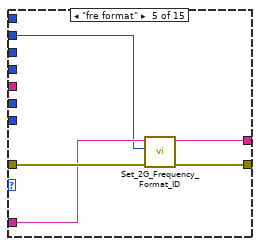
[diagram p12: hidden frame]
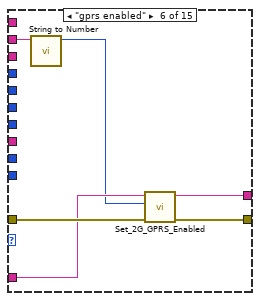
[diagram p13: hidden frame]
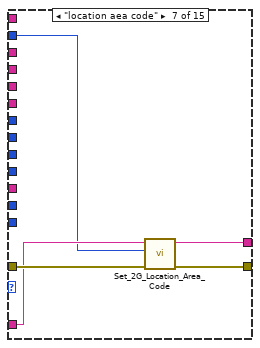
[diagram p14: hidden frame]
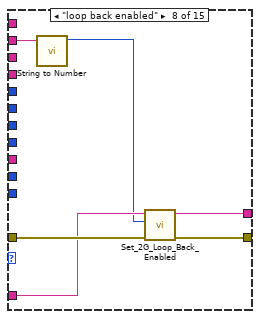
[diagram p15: hidden frame]
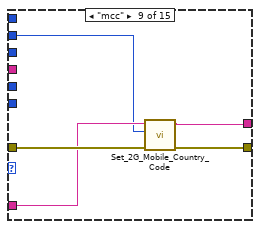
[diagram p16: hidden frame]
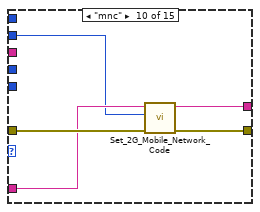
[diagram p17: hidden frame]
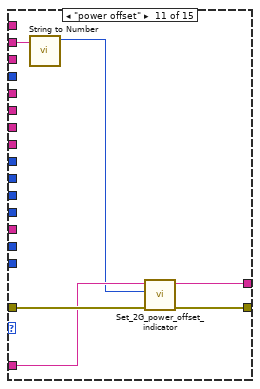
[diagram p18: hidden frame]
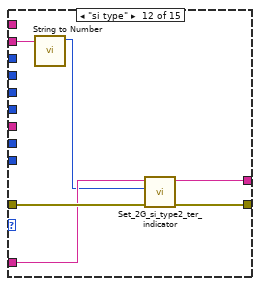
[diagram p19: hidden frame]
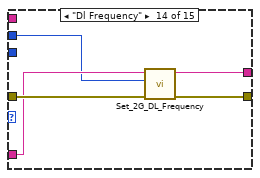
[diagram p20: hidden frame]
diagram:
  n1 = while {
    tunnel: "Band" -> [w11]
    tunnel: "error in" -> [w10]
    tunnel: [w9] -> w3
    tunnel: "Input" -> [w7]
    tunnel: "Base Station" -> [w6]
    stop <- TRUE stop-if-true
    n2 = case shown="\"GSM\"" w11 {
      tunnel: w10 -> [w12 w22 w460 w930]
      tunnel: [w12 w23 w461 w940] -> w9
      tunnel: w7 -> [_ w15 w453 w935]
      tunnel: w6 -> [_ w14 w452 w934]
      frame Default {
      }
      frame "GSM" {
        n3 = Unbundle By Name(w15) -> ("Ref_Cluster.Status"=w13:refnum<vi>, "Ref_Cluster.GSM-PHY"=w16:refnum<vi>, "Ref_Cluster.GSM-CELL"=w17:refnum<vi>, "Ref_Cluster.GSM-GPRS"=w18:refnum<vi>, "Ref_Cluster.GSM-SDR"=w19:refnum<vi>, "Ref_Cluster.GSM-Data"=w21:refnum<vi>)
        n4 = property class="TabCtl (strict)"(reference=w21) -> ("Value"=w20:enum32{"SDR", "CELL", "PHY", "GPRS"})  [unwired: 1 in, 2 out]
        n5 = case shown="\"CELL\"" w20 {
          tunnel: w22 -> [w24 w36 w100 w233 w378]
          tunnel: [w24 w26 w79 w231 w375] -> w23
          tunnel: w19 -> [_ w37 _ _ _]
          tunnel: w18 -> [_ _ _ _ w379]
          tunnel: w17 -> [_ _ w101 _ _]
          tunnel: w16 -> [_ _ _ w234 _]
          tunnel: w15 -> [_ _ _ _ _]
          tunnel: w14 -> [_ w25 w78 w230 w374]
          tunnel: w13 -> [_ w27 w80 w210 w363]
          frame Default {
          }
          frame "SDR" {
            w32 = T9 [enum."Radio Device", enum."Serial name", enum."dl power", enum."ul ref power"] items=["Radio Device", "Serial name", "dl power", "ul ref power"] ("Hardware input")
            n6 = property class="Clust (strict)"(reference=w37, error in=w36) -> (error out=w33:errorcluster, "Value"=w35:T10)  [unwired: 1 out]
            n7 = Unbundle By Name(w35) -> ("Radio Device"=w31:string, "Serial Name"=w30:string, "UL Reference Power"=w34:i32, "DL Reference Power"=w29:i32)
            n8 = for {
              tunnel: w33 -> [w51]
              tunnel: w32 -> [w50] mode=indexing
              tunnel: w25 -> [w49]
              tunnel: T8 "2G" ("Cellular Technology") -> [w40]
              tunnel: w31 -> [w48]
              tunnel: w30 -> [w47]
              tunnel: w34 -> [w45]
              tunnel: w29 -> [w46]
              tunnel: w27 -> [w42]
              tunnel: [w43] -> w26
              tunnel: w25 -> [w41]
              n9 = case shown="\"ul ref power\"" w50 {
                tunnel: w51 -> [w57 w63 w70 w75]
                tunnel: [w56 w62 w69 w74] -> w44
                tunnel: w49 -> [w55 w61 w68 w76]
                tunnel: w40 -> [w54 w60 w67 w77]
                tunnel: w48 -> [w52 _ _ _]
                tunnel: w47 -> [_ w58 _ _]
                tunnel: w46 -> [_ _ w65 _]
                tunnel: w45 -> [_ _ _ w72]
                tunnel: [w53 w59 w66 w73] -> w39
                tunnel: [w52 w58 w64 w71] -> w38
                frame "Radio Device", Default {
                  n10 = call "Set_Radio_Device_Name.vi"("error in (no error)"=w57, "value"=w52, "Cellular Technology"=w54, "Base Station"=w55) -> ("error out"=w56:errorcluster, "Output String"=w53:string)  [unwired: 6 in]
                }
                frame "Serial name" {
                  n11 = call "Set_Radio_Device_Serial_Name.vi"("error in (no error)"=w63, "Serial Name"=w58, "Cellular Technology"=w60, "Base Station"=w61) -> ("error out"=w62:errorcluster, "Output String"=w59:string)  [unwired: 6 in]
                }
                frame "dl power" {
                  n12 = call "Set_Maximum_DL_power.vi"("error in (no error)"=w70, "No of DL antennas Value"=w65, "Cellular Technology"=w67, "Base Station"=w68) -> ("error out"=w69:errorcluster, "Output String"=w66:string)  [unwired: 6 in]
                  n13 = call "Number to String.vi"("DecimaL NU\nmber"=w65) -> ("Decimal String"=w64:string)  [unwired: 10 in]
                }
                frame "ul ref power" {
                  n14 = call "Set_Maximum_UL_Reference_power.vi"("error in (no error)"=w75, "Base Station"=w76, "Cellular Technology"=w77, "No of DL antennas Value"=w72) -> ("error out"=w74:errorcluster, "Output String"=w73:string)  [unwired: 6 in]
                  n15 = call "Number to String.vi"("DecimaL NU\nmber"=w72) -> ("Decimal String"=w71:string)  [unwired: 10 in]
                }
              }
              n16 = call "Status Update.vi"("Base Station"=w41, "Status Reference"=w42, "Band"=w40, "Status"=w39, "Value"=w38, "error in (no error)"=w44) -> ("value out"=w43:errorcluster)  [unwired: 9 in]
            }
          }
          frame "CELL" {
            w81 = T11 [enum."Ul Frequency", enum."Dl Frequency", enum."arfcn", enum."call enables", enum."cell barred access", enum."early classmark sending", enum."fre format", enum."gprs enabled", enum."location aea code", enum."loop back enabled", enum."mcc", enum."mnc", enum."power offset", enum."si type", enum."sms enabled"] items=["Ul Frequency", "Dl Frequency", "Eutra Operating Bands", "arfcn", "call enables", "cell barred access", "early classmark sending", "fre format", "gprs enabled", "location aea code", "loop back enabled", "mcc", "mnc", "power offset", "si type", "sms enabled"] ("cell")
            n17 = property class="Clust (strict)"(reference=w101, error in=w100) -> (error out=w98:errorcluster, "Value"=w99:T12)  [unwired: 1 out]
            n18 = Unbundle By Name(w99) -> ("SMS Enabled"=w97:string, "Eutra Operating Bands"=w95:string, "Power Offset Indicator"=w93:string, "Early Classmark Sending Control"=w94:string, "Location Area Code"=w92:i32, "CALL Enabled"=w91:string, "Loop Back Enabled"=w90:string, "GPRS Enabled"=w89:string, "SI Type 2 ter Indicator"=w88:string, "ARFCN"=w96:i64, "Frequency Format ID"=w87:i64, "Mobile Country Code"=w86:i64, "Mobile Network Code"=w85:i64, "Cell Barred Access"=w84:string, "Downlink Frequency"=w83:i32, "Uplink Frequency"=w82:i32)
            n19 = for {
              tunnel: w78 -> [w125]
              tunnel: w97 -> [w124]
              tunnel: w96 -> [w123]
              tunnel: w95 -> [w122]
              tunnel: w94 -> [w121]
              tunnel: w93 -> [w120]
              tunnel: w92 -> [w119]
              tunnel: w91 -> [w118]
              tunnel: w90 -> [w117]
              tunnel: w89 -> [w116]
              tunnel: w88 -> [w115]
              tunnel: w87 -> [w114]
              tunnel: w86 -> [w113]
              tunnel: w85 -> [w112]
              tunnel: w84 -> [w111]
              tunnel: w83 -> [w110]
              tunnel: w82 -> [w109]
              tunnel: w98 -> [w126]
              tunnel: w81 -> [w108] mode=indexing
              tunnel: w80 -> [w105]
              tunnel: [w106] -> w79
              tunnel: w78 -> [w102]
              n20 = case shown="\"sms enabled\"" w108 {
                tunnel: w126 -> [w131 w137 w143 w149 w154 w160 w165 w171 w176 w181 w187 w193 w199 w204 w209]
                tunnel: [w130 w136 w142 w148 w153 w159 w164 w170 w175 w180 w186 w192 w198 w203 w208] -> w107
                tunnel: w125 -> [w129 w135 w141 w147 w152 w158 w163 w169 w174 w179 w185 w191 w196 w202 w207]
                tunnel: w124 -> [_ _ _ _ _ _ _ _ _ _ _ _ w197 _ _]
                tunnel: w123 -> [w128 _ _ _ _ _ _ _ _ _ _ _ _ _ _]
                tunnel: w122 -> [_ _ _ _ _ _ _ _ _ _ _ _ _ _ _]
                tunnel: w121 -> [_ _ _ w146 _ _ _ _ _ _ _ _ _ _ _]
                tunnel: w120 -> [_ _ _ _ _ _ _ _ _ _ w184 _ _ _ _]
                tunnel: w119 -> [_ _ _ _ _ _ w162 _ _ _ _ _ _ _ _]
                tunnel: w118 -> [_ w134 _ _ _ _ _ _ _ _ _ _ _ _ _]
                tunnel: w117 -> [_ _ _ _ _ _ _ w168 _ _ _ _ _ _ _]
                tunnel: w116 -> [_ _ _ _ _ w157 _ _ _ _ _ _ _ _ _]
                tunnel: w115 -> [_ _ _ _ _ _ _ _ _ _ _ w190 _ _ _]
                tunnel: w114 -> [_ _ _ _ w151 _ _ _ _ _ _ _ _ _ _]
                tunnel: w113 -> [_ _ _ _ _ _ _ _ w173 _ _ _ _ _ _]
                tunnel: w112 -> [_ _ _ _ _ _ _ _ _ w178 _ _ _ _ _]
                tunnel: w111 -> [_ _ w140 _ _ _ _ _ _ _ _ _ _ _ _]
                tunnel: w110 -> [_ _ _ _ _ _ _ _ _ _ _ _ _ w201 _]
                tunnel: w109 -> [_ _ _ _ _ _ _ _ _ _ _ _ _ _ w206]
                tunnel: [w127 w132 w138 w144 w150 w155 w161 w166 w172 w177 w182 w188 w194 w200 w205] -> w104
                frame "arfcn", Default {
                  n21 = call "Set_2G_ARFCN.vi"("error in (no error)"=w131, "value"=w128, "Base Station"=w129) -> ("error out"=w130:errorcluster, "Output String"=w127:string)  [unwired: 7 in]
                }
                frame "call enables" {
                  n22 = call "String to Number.vi"("Decimal String"=w134) -> ("Decimal Number"=w133:i32)  [unwired: 10 in]
                  n23 = call "Set_2G_Call_Enabled.vi"("error in (no error)"=w137, "value"=w133, "Base Station"=w135) -> ("error out"=w136:errorcluster, "Output String"=w132:string)  [unwired: 7 in]
                }
                frame "cell barred access" {
                  n24 = call "String to Number.vi"("Decimal String"=w140) -> ("Decimal Number"=w139:i32)  [unwired: 10 in]
                  n25 = call "Set_2G_Cell_Barred_Access.vi"("error in (no error)"=w143, "value"=w139, "Base Station"=w141) -> ("error out"=w142:errorcluster, "Output String"=w138:string)  [unwired: 7 in]
                }
                frame "early classmark sending" {
                  n26 = call "String to Number.vi"("Decimal String"=w146) -> ("Decimal Number"=w145:i32)  [unwired: 10 in]
                  n27 = call "Set_2G_Early_Classmark_Sending_Control.vi"("error in (no error)"=w149, "value"=w145, "Base Station"=w147) -> ("error out"=w148:errorcluster, "Output String"=w144:string)  [unwired: 7 in]
                }
                frame "fre format" {
                  n28 = call "Set_2G_Frequency_Format_ID.vi"("error in (no error)"=w154, "value"=w151, "Base Station"=w152) -> ("error out"=w153:errorcluster, "Output String"=w150:string)  [unwired: 7 in]
                }
                frame "gprs enabled" {
                  n29 = call "String to Number.vi"("Decimal String"=w157) -> ("Decimal Number"=w156:i32)  [unwired: 10 in]
                  n30 = call "Set_2G_GPRS_Enabled.vi"("error in (no error)"=w160, "value"=w156, "Base Station"=w158) -> ("error out"=w159:errorcluster, "Output String"=w155:string)  [unwired: 7 in]
                }
                frame "location aea code" {
                  n31 = call "Set_2G_Location_Area_Code.vi"("error in (no error)"=w165, "value"=w162, "Base Station"=w163) -> ("error out"=w164:errorcluster, "Output String"=w161:string)  [unwired: 7 in]
                }
                frame "loop back enabled" {
                  n32 = call "String to Number.vi"("Decimal String"=w168) -> ("Decimal Number"=w167:i32)  [unwired: 10 in]
                  n33 = call "Set_2G_Loop_Back_Enabled.vi"("error in (no error)"=w171, "value"=w167, "Base Station"=w169) -> ("error out"=w170:errorcluster, "Output String"=w166:string)  [unwired: 7 in]
                }
                frame "mcc" {
                  n34 = call "Set_2G_Mobile_Country_Code.vi"("error in (no error)"=w176, "value"=w173, "Base Station"=w174) -> ("error out"=w175:errorcluster, "Output String"=w172:string)  [unwired: 7 in]
                }
                frame "mnc" {
                  n35 = call "Set_2G_Mobile_Network_Code.vi"("error in (no error)"=w181, "value"=w178, "Base Station"=w179) -> ("error out"=w180:errorcluster, "Output String"=w177:string)  [unwired: 7 in]
                }
                frame "power offset" {
                  n36 = call "String to Number.vi"("Decimal String"=w184) -> ("Decimal Number"=w183:i32)  [unwired: 10 in]
                  n37 = call "Set_2G_power_offset_indicator.vi"("error in (no error)"=w187, "value"=w183, "Base Station"=w185) -> ("error out"=w186:errorcluster, "Output String"=w182:string)  [unwired: 7 in]
                }
                frame "si type" {
                  n38 = call "String to Number.vi"("Decimal String"=w190) -> ("Decimal Number"=w189:i32)  [unwired: 10 in]
                  n39 = call "Set_2G_si_type2_ter_indicator.vi"("error in (no error)"=w193, "value"=w189, "Base Station"=w191) -> ("error out"=w192:errorcluster, "Output String"=w188:string)  [unwired: 7 in]
                }
                frame "sms enabled" {
                  n40 = call "String to Number.vi"("Decimal String"=w197) -> ("Decimal Number"=w195:i32)  [unwired: 10 in]
                  n41 = call "Set_2G_SMS_Enabled.vi"("error in (no error)"=w199, "value"=w195, "Base Station"=w196) -> ("error out"=w198:errorcluster, "Output String"=w194:string)  [unwired: 7 in]
                }
                frame "Dl Frequency" {
                  n42 = call "Set_2G_DL_Frequency.vi"("error in (no error)"=w204, "value"=w201, "Base Station"=w202) -> ("error out"=w203:errorcluster, "Output String"=w200:string)  [unwired: 7 in]
                }
                frame "Ul Frequency" {
                  n43 = call "Set_2G_SMS_Enabled.vi"("error in (no error)"=w209, "value"=w206, "Base Station"=w207) -> ("error out"=w208:errorcluster, "Output String"=w205:string)  [unwired: 7 in]
                }
              }
              n44 = call "Status Update.vi"("Base Station"=w102, "Status Reference"=w105, "Band"="2G", "Status"=w104, "error in (no error)"=w107) -> ("value out"=w106:errorcluster)  [unwired: 10 in]
            }
          }
          frame "PHY" {
            w211 = T13 [enum."RAch maxi retranmission", enum."rach transmission slots", enum."rach call", enum."Rach access control access", enum."block for acs", enum."multiframe forpg", enum."pow con indi", enum."radio link timout", enum."cell reselect", enum."attach detach", enum."ccch", enum."t3212", enum."dtx", enum."pow contro level", enum."min received sig", enum."hal rate", enum."add reselect"] items=["ccch", "add reselect", "attach detach", "block for acs", "cell reselect", "dtx", "hal rate", "min received sig", "multiframe forpg", "pow con indi", "pow contro level", "Rach access control access", "rach call", "RAch maxi retranmission", "rach transmission slots", "radio link timout", "t3212"] ("Phy")
            n45 = property class="Clust (strict)"(reference=w234, error in=w233) -> (error out=w232:errorcluster, "Value"=w229:T14)  [unwired: 1 out]
            n46 = Unbundle By Name(w229) -> ("RACH Maximum Retransmission"=w216:string, "RACH Transmission Slots"=w215:string, "RACH Call Reestablishment"=w217:string, "RACH Access Control Class"=w218:string, "Block for Access Grant"=w225:string, "Multiframe for Paging"=w221:string, "Power Control Indicator"=w220:string, "Radio Link Timeout"=w214:string, "Cell Reselect Hysterisis"=w212:string, "Attach/Detach Allowed"=w226:string, "CCCH Combinations"=w228:string, "t3212"=w213:i64, "DTX Indicator"=w224:string, "Power Control Level"=w219:i64, "Minimum Received Signal Level"=w222:i64, "Half Rate Support"=w223:string, "Add Reselect"=w227:string)
            n47 = for {
              tunnel: w230 -> [w238]
              tunnel: w228 -> [w258]
              tunnel: w227 -> [w257]
              tunnel: w226 -> [w256]
              tunnel: w225 -> [w255]
              tunnel: w224 -> [w254]
              tunnel: w223 -> [w253]
              tunnel: w222 -> [w252]
              tunnel: w221 -> [w251]
              tunnel: w220 -> [w250]
              tunnel: w219 -> [w249]
              tunnel: w218 -> [w248]
              tunnel: w217 -> [w247]
              tunnel: w216 -> [w246]
              tunnel: w215 -> [w245]
              tunnel: w214 -> [w244]
              tunnel: w213 -> [w243]
              tunnel: w212 -> [w242]
              tunnel: w211 -> [w241] mode=indexing
              tunnel: w232 -> [w260]
              tunnel: [w240] -> w231
              tunnel: w210 -> [w239]
              n48 = case shown="\"t3212\"" w241 {
                tunnel: w260 -> [w264 w272 w278 w284 w290 w296 w302 w308 w312 w320 w326 w332 w338 w344 w350 w356 w362]
                tunnel: [w266 w271 w277 w283 w289 w295 w301 w307 w314 w319 w325 w331 w337 w342 w349 w355 w361] -> w259
                tunnel: w238 -> [w265 w270 w276 w282 w288 w294 w300 w306 w313 w318 w324 w330 w336 w343 w348 w354 w360]
                tunnel: w258 -> [w261 _ _ _ _ _ _ _ _ _ _ _ _ _ _ _ _]
                tunnel: w257 -> [_ w267 _ _ _ _ _ _ _ _ _ _ _ _ _ _ _]
                tunnel: w256 -> [_ _ w273 _ _ _ _ _ _ _ _ _ _ _ _ _ _]
                tunnel: w255 -> [_ _ _ w280 _ _ _ _ _ _ _ _ _ _ _ _ _]
                tunnel: w254 -> [_ _ _ _ _ w291 _ _ _ _ _ _ _ _ _ _ _]
                tunnel: w253 -> [_ _ _ _ _ _ w297 _ _ _ _ _ _ _ _ _ _]
                tunnel: w252 -> [_ _ _ _ _ _ _ w303 _ _ _ _ _ _ _ _ _]
                tunnel: w251 -> [_ _ _ _ _ _ _ _ w309 _ _ _ _ _ _ _ _]
                tunnel: w250 -> [_ _ _ _ _ _ _ _ _ w315 _ _ _ _ _ _ _]
                tunnel: w249 -> [_ _ _ _ _ _ _ _ _ _ w321 _ _ _ _ _ _]
                tunnel: w248 -> [_ _ _ _ _ _ _ _ _ _ _ w327 _ _ _ _ _]
                tunnel: w247 -> [_ _ _ _ _ _ _ _ _ _ _ _ w333 _ _ _ _]
                tunnel: w246 -> [_ _ _ _ _ _ _ _ _ _ _ _ _ w339 _ _ _]
                tunnel: w245 -> [_ _ _ _ _ _ _ _ _ _ _ _ _ _ w345 _ _]
                tunnel: w244 -> [_ _ _ _ _ _ _ _ _ _ _ _ _ _ _ w351 _]
                tunnel: w243 -> [_ _ _ _ _ _ _ _ _ _ _ _ _ _ _ _ w357]
                tunnel: w242 -> [_ _ _ _ w285 _ _ _ _ _ _ _ _ _ _ _ _]
                tunnel: [w262 w268 w274 w279 w286 w292 w298 w305 w310 w316 w323 w328 w334 w340 w346 w352 w359] -> w236
                tunnel: [w261 w267 w273 w280 w285 w291 w297 w304 w309 w315 w322 w327 w333 w339 w345 w351 w358] -> w235
                frame "ccch", Default {
                  n49 = call "String to Number.vi"("Decimal String"=w261) -> ("Decimal Number"=w263:i32)  [unwired: 10 in]
                  n50 = call "Set 2G CCCH Combination.vi"("error in (no error)"=w264, "value"=w263, "Base Station"=w265) -> ("error out"=w266:errorcluster, "Output String"=w262:string)  [unwired: 7 in]
                }
                frame "add reselect" {
                  n51 = call "String to Number.vi"("Decimal String"=w267) -> ("Decimal Number"=w269:i32)  [unwired: 10 in]
                  n52 = call "Set_2G_Add_Reselect_Indicator.vi"("error in (no error)"=w272, "value"=w269, "Base Station"=w270) -> ("error out"=w271:errorcluster, "Output String"=w268:string)  [unwired: 7 in]
                }
                frame "attach detach" {
                  n53 = call "String to Number.vi"("Decimal String"=w273) -> ("Decimal Number"=w275:i32)  [unwired: 10 in]
                  n54 = call "Set_2G_Attach_Detach_Allowed.vi"("error in (no error)"=w278, "value"=w275, "Base Station"=w276) -> ("error out"=w277:errorcluster, "Output String"=w274:string)  [unwired: 7 in]
                }
                frame "block for acs" {
                  n55 = call "String to Number.vi"("Decimal String"=w280) -> ("Decimal Number"=w281:i32)  [unwired: 10 in]
                  n56 = call "Set_2G_Block_For_Access_Grant.vi"("error in (no error)"=w284, "value"=w281, "Base Station"=w282) -> ("error out"=w283:errorcluster, "Output String"=w279:string)  [unwired: 7 in]
                }
                frame "cell reselect" {
                  n57 = call "String to Number.vi"("Decimal String"=w285) -> ("Decimal Number"=w287:i32)  [unwired: 10 in]
                  n58 = call "Set_2G_Cell_Reselect_Hysteresis.vi"("error in (no error)"=w290, "value"=w287, "Base Station"=w288) -> ("error out"=w289:errorcluster, "Output String"=w286:string)  [unwired: 7 in]
                }
                frame "dtx" {
                  n59 = call "String to Number.vi"("Decimal String"=w291) -> ("Decimal Number"=w293:i32)  [unwired: 10 in]
                  n60 = call "Set_2G_DTX_Indicator.vi"("error in (no error)"=w296, "value"=w293, "Base Station"=w294) -> ("error out"=w295:errorcluster, "Output String"=w292:string)  [unwired: 7 in]
                }
                frame "hal rate" {
                  n61 = call "String to Number.vi"("Decimal String"=w297) -> ("Decimal Number"=w299:i32)  [unwired: 10 in]
                  n62 = call "Set_2G_Half_Rate_Support.vi"("error in (no error)"=w302, "value"=w299, "Base Station"=w300) -> ("error out"=w301:errorcluster, "Output String"=w298:string)  [unwired: 7 in]
                }
                frame "min received sig" {
                  n63 = call "Set_2G_Minimum_Received_Signal_Level.vi"("error in (no error)"=w308, "value"=w303, "Base Station"=w306) -> ("error out"=w307:errorcluster, "Output String"=w305:string)  [unwired: 7 in]
                  n64 = call "Number to String.vi"("DecimaL NU\nmber"=w303) -> ("Decimal String"=w304:string)  [unwired: 10 in]
                }
                frame "multiframe forpg" {
                  n65 = call "String to Number.vi"("Decimal String"=w309) -> ("Decimal Number"=w311:i32)  [unwired: 10 in]
                  n66 = call "Set_2G_Multiframe_For_Paging.vi"("error in (no error)"=w312, "value"=w311, "Base Station"=w313) -> ("error out"=w314:errorcluster, "Output String"=w310:string)  [unwired: 7 in]
                }
                frame "pow con indi" {
                  n67 = call "String to Number.vi"("Decimal String"=w315) -> ("Decimal Number"=w317:i32)  [unwired: 10 in]
                  n68 = call "Set_2G_Power_Control_Indicator.vi"("error in (no error)"=w320, "value"=w317, "Base Station"=w318) -> ("error out"=w319:errorcluster, "Output String"=w316:string)  [unwired: 7 in]
                }
                frame "pow contro level" {
                  n69 = call "Set_2G_Power_Control_Level .vi"("error in (no error)"=w326, "value"=w321, "Base Station"=w324) -> ("error out"=w325:errorcluster, "Output String"=w323:string)  [unwired: 7 in]
                  n70 = call "Number to String.vi"("DecimaL NU\nmber"=w321) -> ("Decimal String"=w322:string)  [unwired: 10 in]
                }
                frame "Rach access control access" {
                  n71 = call "String to Number.vi"("Decimal String"=w327) -> ("Decimal Number"=w329:i32)  [unwired: 10 in]
                  n72 = call "Set_2G_RACH_Access_Control_Class.vi"("error in (no error)"=w332, "value"=w329, "Base Station"=w330) -> ("error out"=w331:errorcluster, "Output String"=w328:string)  [unwired: 7 in]
                }
                frame "rach call" {
                  n73 = call "String to Number.vi"("Decimal String"=w333) -> ("Decimal Number"=w335:i32)  [unwired: 10 in]
                  n74 = call "Set_2G_RACH_Call_Reestablishment.vi"("error in (no error)"=w338, "value"=w335, "Base Station"=w336) -> ("error out"=w337:errorcluster, "Output String"=w334:string)  [unwired: 7 in]
                }
                frame "RAch maxi retranmission" {
                  n75 = call "String to Number.vi"("Decimal String"=w339) -> ("Decimal Number"=w341:i32)  [unwired: 10 in]
                  n76 = call "Set_2G_RACH_Maximum_Retransmission.vi"("error in (no error)"=w344, "value"=w341, "Base Station"=w343) -> ("error out"=w342:errorcluster, "Output String"=w340:string)  [unwired: 7 in]
                }
                frame "rach transmission slots" {
                  n77 = call "String to Number.vi"("Decimal String"=w345) -> ("Decimal Number"=w347:i32)  [unwired: 10 in]
                  n78 = call "Set_2G_RACH_Transmission_Slots.vi"("error in (no error)"=w350, "value"=w347, "Base Station"=w348) -> ("error out"=w349:errorcluster, "Output String"=w346:string)  [unwired: 7 in]
                }
                frame "radio link timout" {
                  n79 = call "String to Number.vi"("Decimal String"=w351) -> ("Decimal Number"=w353:i32)  [unwired: 10 in]
                  n80 = call "Set_2G_Radio_Link_Timeout.vi"("error in (no error)"=w356, "value"=w353, "Base Station"=w354) -> ("error out"=w355:errorcluster, "Output String"=w352:string)  [unwired: 7 in]
                }
                frame "t3212" {
                  n81 = call "Set_2G_t3212.vi"("error in (no error)"=w362, "value"=w357, "Base Station"=w360) -> ("error out"=w361:errorcluster, "Output String"=w359:string)  [unwired: 7 in]
                  n82 = call "Number to String.vi"("DecimaL NU\nmber"=w357) -> ("Decimal String"=w358:string)  [unwired: 10 in]
                }
              }
              n83 = call "Status Update.vi"("Base Station"=w238, "Status Reference"=w239, "Band"="2G", "Status"=w236, "Value"=w235, "error in (no error)"=w259) -> ("value out"=w240:errorcluster)  [unwired: 9 in]
            }
          }
          frame "GPRS" {
            w364 = T15 [enum."priority access", enum."access burst", enum."nack countdown", enum."bcch pdch", enum."rac", enum."network control", enum."t3168", enum."t3192", enum."gprs parameter alpha"] items=["bcch pdch", "gprs parameter alpha", "access burst", "nack countdown", "network control", "priority access", "rac", "t3168", "t3192"] ("gprs")
            n84 = property class="Clust (strict)"(reference=w379, error in=w378) -> (error out=w376:errorcluster, "Value"=w377:T16)  [unwired: 1 out]
            n85 = Unbundle By Name(w377) -> ("Priority Access THR"=w369:string, "Acess Burst Type"=w371:string, "Nack Countdown"=w365:string, "BCCH/PDCH Measurement"=w373:string, "Routing Area Code(RAC)"=w368:i32, "Network Control Order"=w370:string, "t3168"=w367:string, "t3192"=w366:string, "Alpha"=w372:string)
            n86 = for {
              tunnel: w374 -> [w383]
              tunnel: w373 -> [w395]
              tunnel: w372 -> [w394]
              tunnel: w371 -> [w393]
              tunnel: w370 -> [w392]
              tunnel: w369 -> [w391]
              tunnel: w368 -> [w390]
              tunnel: w367 -> [w389]
              tunnel: w366 -> [w388]
              tunnel: w365 -> [w387]
              tunnel: w364 -> [w386] mode=indexing
              tunnel: w376 -> [w397]
              tunnel: [w385] -> w375
              tunnel: w363 -> [w384]
              n87 = case shown="\"rac\"" w386 {
                tunnel: w397 -> [w403 w409 w414 w420 w426 w432 w438 w444 w450]
                tunnel: [w402 w408 w413 w419 w425 w431 w437 w443 w449] -> w396
                tunnel: w383 -> [w401 w407 w412 w418 w424 w430 w436 w442 w448]
                tunnel: w395 -> [w398 _ _ _ _ _ _ _ _]
                tunnel: w394 -> [_ w404 _ _ _ _ _ _ _]
                tunnel: w393 -> [_ _ w410 _ _ _ _ _ _]
                tunnel: w392 -> [_ _ _ _ w421 _ _ _ _]
                tunnel: w391 -> [_ _ _ _ _ w427 _ _ _]
                tunnel: w390 -> [_ _ _ _ _ _ w435 _ _]
                tunnel: w389 -> [_ _ _ _ _ _ _ w440 _]
                tunnel: w388 -> [_ _ _ _ _ _ _ _ w446]
                tunnel: w387 -> [_ _ _ w415 _ _ _ _ _]
                tunnel: [w399 w405 w411 w416 w422 w428 w434 w439 w445] -> w381
                tunnel: [w398 w404 w410 w415 w421 w427 w433 w440 w446] -> w380
                frame "bcch pdch", Default {
                  n88 = call "String to Number.vi"("Decimal String"=w398) -> ("Decimal Number"=w400:i32)  [unwired: 10 in]
                  n89 = call "Set_2G_GPRS _BCCH_PDCH_Measurement.vi"("error in (no error)"=w403, "value"=w400, "Base Station"=w401) -> ("error out"=w402:errorcluster, "Output String"=w399:string)  [unwired: 7 in]
                }
                frame "gprs parameter alpha" {
                  n90 = call "String to Number.vi"("Decimal String"=w404) -> ("Decimal Number"=w406:i32)  [unwired: 10 in]
                  n91 = call "Set_2G_GPRS_Parameter_Alpha.vi"("error in (no error)"=w409, "value"=w406, "Base Station"=w407) -> ("error out"=w408:errorcluster, "Output String"=w405:string)  [unwired: 7 in]
                }
                frame "access burst" {
                  n92 = call "Set_GPRS_Access_Burst_Type.vi"("error in (no error)"=w414, "value"=w410, "Base Station"=w412) -> ("error out"=w413:errorcluster, "Output String"=w411:string)  [unwired: 7 in]
                }
                frame "nack countdown" {
                  n93 = call "String to Number.vi"("Decimal String"=w415) -> ("Decimal Number"=w417:i32)  [unwired: 10 in]
                  n94 = call "Set_GPRS_NACK_Countdown.vi"("error in (no error)"=w420, "value"=w417, "Base Station"=w418) -> ("error out"=w419:errorcluster, "Output String"=w416:string)  [unwired: 7 in]
                }
                frame "network control" {
                  n95 = call "String to Number.vi"("Decimal String"=w421) -> ("Decimal Number"=w423:i32)  [unwired: 10 in]
                  n96 = call "Set_GPRS_Network_Control_Order.vi"("error in (no error)"=w426, "value"=w423, "Base Station"=w424) -> ("error out"=w425:errorcluster, "Output String"=w422:string)  [unwired: 7 in]
                }
                frame "priority access" {
                  n97 = call "String to Number.vi"("Decimal String"=w427) -> ("Decimal Number"=w429:i32)  [unwired: 10 in]
                  n98 = call "Set_GPRS_Priority_Access_THR.vi"("error in (no error)"=w432, "value"=w429, "Base Station"=w430) -> ("error out"=w431:errorcluster, "Output String"=w428:string)  [unwired: 7 in]
                }
                frame "rac" {
                  n99 = call "Number to String.vi"("DecimaL NU\nmber"=w435) -> ("Decimal String"=w433:string)  [unwired: 10 in]
                  n100 = call "Set_GPRS_RAC.vi"("error in (no error)"=w438, "value"=w433, "Base Station"=w436) -> ("error out"=w437:errorcluster, "Output String"=w434:string)  [unwired: 7 in]
                }
                frame "t3168" {
                  n101 = call "String to Number.vi"("Decimal String"=w440) -> ("Decimal Number"=w441:i32)  [unwired: 10 in]
                  n102 = call "Set_GPRS_t3168.vi"("error in (no error)"=w444, "value"=w441, "Base Station"=w442) -> ("error out"=w443:errorcluster, "Output String"=w439:string)  [unwired: 7 in]
                }
                frame "t3192" {
                  n103 = call "String to Number.vi"("Decimal String"=w446) -> ("Decimal Number"=w447:i32)  [unwired: 10 in]
                  n104 = call "Set_GPRS_t3192.vi"("error in (no error)"=w450, "value"=w447, "Base Station"=w448) -> ("error out"=w449:errorcluster, "Output String"=w445:string)  [unwired: 7 in]
                }
              }
              n105 = call "Status Update.vi"("Base Station"=w383, "Status Reference"=w384, "Band"="2G", "Status"=w381, "Value"=w380, "error in (no error)"=w396) -> ("value out"=w385:errorcluster)  [unwired: 9 in]
            }
          }
        }
      }
      frame "eNodeB" {
        n106 = Unbundle By Name(w453) -> ("Ref_Cluster.Status"=w451:refnum<vi>, "Ref_Cluster.LTE-PHY"=w454:refnum<vi>, "Ref_Cluster.LTE-CELL"=w455:refnum<vi>, "Ref_Cluster.LTE-RRC"=w456:refnum<vi>, "Ref_Cluster.LTE-SDR"=w457:refnum<vi>, "Ref_Cluster.eNodeB-Data"=w459:refnum<vi>)
        n107 = property class="TabCtl (strict)"(reference=w459) -> ("Value"=w458:enum32{"SDR", "CELL", "PHY", "RRC"})  [unwired: 1 in, 2 out]
        n108 = case shown="\"CELL\"" w458 {
          tunnel: w460 -> [w462 w476 w554 w689 w877]
          tunnel: [w462 w471 w536 w660 w874] -> w461
          tunnel: w457 -> [_ w477 _ _ _]
          tunnel: w456 -> [_ _ _ _ w878]
          tunnel: w455 -> [_ _ w555 _ _]
          tunnel: w454 -> [_ _ _ w690 _]
          tunnel: w453 -> [_ _ _ _ _]
          tunnel: w452 -> [_ w470 w551 w688 w873]
          tunnel: w451 -> [_ w463 w534 w658 w865]
          frame Default {
          }
          frame "SDR" {
            w472 = T17 [enum."Radio Device", enum."Serial name", enum."dl power", enum."ul ref power", enum."Ul Antennas", enum."Dl Antennas"] items=["Radio Device", "Serial name", "dl power", "ul ref power", "Ul Antennas", "Dl Antennas"] ("Hardware input")
            n109 = property class="Clust (strict)"(reference=w477, error in=w476) -> (error out=w473:errorcluster, "Value"=w475:T18)  [unwired: 1 out]
            n110 = Unbundle By Name(w475) -> ("UL Antennas"=w464:string, "DL Antennas"=w465:string, "Radio Device"=w469:string, "Serail Name"=w468:string, "UL Reference Power"=w474:i32, "DL Reference Power"=w467:i32)
            n111 = for {
              tunnel: w473 -> [w493]
              tunnel: w472 -> [w492] mode=indexing
              tunnel: [w483] -> w471
              tunnel: w470 -> [w481]
              tunnel: T8 "4G" ("Cellular Technology") -> [w490]
              tunnel: w469 -> [w489]
              tunnel: w468 -> [w488]
              tunnel: w474 -> [w486]
              tunnel: w467 -> [w487]
              tunnel: w465 -> [w485]
              tunnel: w464 -> [w484]
              tunnel: w463 -> [w482]
              n112 = case shown="\"ul ref power\"" w492 {
                tunnel: w493 -> [w499 w505 w512 w517 w524 w531]
                tunnel: [w498 w504 w511 w516 w523 w530] -> w491
                tunnel: w481 -> [w497 w503 w510 w518 w525 w532]
                tunnel: w490 -> [w496 w502 w509 w519 w526 w533]
                tunnel: w489 -> [w494 _ _ _ _ _]
                tunnel: w488 -> [_ w500 _ _ _ _]
                tunnel: w487 -> [_ _ w507 _ _ _]
                tunnel: w486 -> [_ _ _ w515 _ _]
                tunnel: w485 -> [_ _ _ _ _ w528]
                tunnel: w484 -> [_ _ _ _ w520 _]
                tunnel: [w495 w501 w508 w513 w521 w527] -> w479
                tunnel: [w494 w500 w506 w514 w520 w528] -> w478
                frame "Radio Device", Default {
                  n113 = call "Set_Radio_Device_Name.vi"("error in (no error)"=w499, "value"=w494, "Cellular Technology"=w496, "Base Station"=w497) -> ("error out"=w498:errorcluster, "Output String"=w495:string)  [unwired: 6 in]
                }
                frame "Serial name" {
                  n114 = call "Set_Radio_Device_Serial_Name.vi"("error in (no error)"=w505, "Serial Name"=w500, "Cellular Technology"=w502, "Base Station"=w503) -> ("error out"=w504:errorcluster, "Output String"=w501:string)  [unwired: 6 in]
                }
                frame "dl power" {
                  n115 = call "Number to String.vi"("DecimaL NU\nmber"=w507) -> ("Decimal String"=w506:string)  [unwired: 10 in]
                  n116 = call "Set_Maximum_DL_power.vi"("error in (no error)"=w512, "No of DL antennas Value"=w507, "Cellular Technology"=w509, "Base Station"=w510) -> ("error out"=w511:errorcluster, "Output String"=w508:string)  [unwired: 6 in]
                }
                frame "ul ref power" {
                  n117 = call "Set_Maximum_UL_Reference_power.vi"("error in (no error)"=w517, "Base Station"=w518, "Cellular Technology"=w519, "No of DL antennas Value"=w515) -> ("error out"=w516:errorcluster, "Output String"=w513:string)  [unwired: 6 in]
                  n118 = call "Number to String.vi"("DecimaL NU\nmber"=w515) -> ("Decimal String"=w514:string)  [unwired: 10 in]
                }
                frame "Ul Antennas" {
                  n119 = call "String to Number.vi"("Decimal String"=w520) -> ("Decimal Number"=w522:i32)  [unwired: 10 in]
                  n120 = call "Set_Number_of_UL_Antennas.vi"("error in (no error)"=w524, "No of UL antennas Value"=w522, "Cellular Technology"=w526, "Base Station"=w525) -> ("error out"=w523:errorcluster, "Output String"=w521:string)  [unwired: 6 in]
                }
                frame "Dl Antennas" {
                  n121 = call "String to Number.vi"("Decimal String"=w528) -> ("Decimal Number"=w529:i32)  [unwired: 10 in]
                  n122 = call "Set_Number_of_DL_Antennas.vi"("error in (no error)"=w531, "No of DL antennas Value"=w529, "Cellular Technology"=w533, "Base Station"=w532) -> ("error out"=w530:errorcluster, "Output String"=w527:string)  [unwired: 6 in]
                }
              }
              n123 = call "Status Update.vi"("Base Station"=w481, "Status Reference"=w482, "Band"="4G", "Status"=w479, "Value"=w478, "error in (no error)"=w491) -> ("value out"=w483:errorcluster)  [unwired: 9 in]
            }
          }
          frame "CELL" {
            w535 = T19 [enum."Duplex Mode", enum."Eutra operating band", enum."Measurement report", enum."Carrier BW", enum."Physical Cell ID", enum."network name", enum."DL Frequency", enum."IMS Enable", enum."Transmission Mode", enum."MNC length", enum."MCC", enum."IMS Enable"] items=["Carrier BW", "DL Frequency", "Duplex Mode", "Eutra operating band", "Measurement report", "MNC length", "MCC", "MNC", "network name", "Physical Cell ID", "Tracking area code", "Transmission Mode", "IMS Enable", "UL frequency"] ("cell")
            n124 = property class="Clust (strict)"(reference=w555, error in=w554) -> (error out=w552:errorcluster, "Value"=w553:T20)  [unwired: 1 out]
            n125 = Unbundle By Name(w553) -> ("Duplex Mode"=w550:string, "Eutra Operating Bands"=w548:string, "Measurement Report"=w546:string, "Carrier Bandwidth"=w547:string, "Physical Cell ID"=w545:i64, "Network Name"=w544:string, "DL Frequency"=w543:i32, "UL Frequency"=w542:i32, "Transmission Mode"=w541:string, "MNC Length"=w549:string, "IMS Enabled"=w540:string, "Tracking Area Code"=w539:i32, "Mobile Country Code"=w538:i32, "Mobile Network Code"=w537:i32)
            n126 = for {
              tunnel: w551 -> [w557]
              tunnel: w550 -> [w572]
              tunnel: w549 -> [w569]
              tunnel: w548 -> [w571]
              tunnel: w547 -> [w575]
              tunnel: w546 -> [w570]
              tunnel: w545 -> [w565]
              tunnel: w544 -> [w566]
              tunnel: w543 -> [w573]
              tunnel: w542 -> [w562]
              tunnel: w541 -> [w563]
              tunnel: w540 -> [w574]
              tunnel: w539 -> [w564]
              tunnel: w538 -> [w568]
              tunnel: w537 -> [w567]
              tunnel: w552 -> [w577]
              tunnel: [w561] -> w536
              tunnel: w535 -> [w576] mode=indexing
              tunnel: w534 -> [w560]
              n127 = case shown="\"Eutra operating band\"" w576 {
                tunnel: w577 -> [w583 w588 w594 w599 w604 w611 w618 w624 w630 w634 w640 w646 w651 w657]
                tunnel: w557 -> [w582 w587 w593 w598 w603 w610 w617 w623 w629 _ w639 w645 w650 w656]
                tunnel: [w581 w586 w592 w597 w602 w609 w616 w622 w628 w633 w638 w644 w649 w655] -> w578
                tunnel: w575 -> [w580 _ _ _ _ _ _ _ _ _ _ _ _ _]
                tunnel: w574 -> [_ w584 _ _ _ _ _ _ _ _ _ _ _ _]
                tunnel: w573 -> [_ _ w590 _ _ _ _ _ _ _ _ _ _ _]
                tunnel: w572 -> [_ _ _ w596 _ _ _ _ _ _ _ _ _ _]
                tunnel: w571 -> [_ _ _ _ w601 _ _ _ _ _ _ _ _ _]
                tunnel: w570 -> [_ _ _ _ _ w608 _ _ _ _ _ _ _ _]
                tunnel: w569 -> [_ _ _ _ _ _ w615 _ _ _ _ _ _ _]
                tunnel: w568 -> [_ _ _ _ _ _ _ w621 _ _ _ _ _ _]
                tunnel: w567 -> [_ _ _ _ _ _ _ _ w627 _ _ _ _ _]
                tunnel: w566 -> [_ _ _ _ _ _ _ _ _ w631 _ _ _ _]
                tunnel: w565 -> [_ _ _ _ _ _ _ _ _ _ w636 _ _ _]
                tunnel: w564 -> [_ _ _ _ _ _ _ _ _ _ _ w641 _ _]
                tunnel: w563 -> [_ _ _ _ _ _ _ _ _ _ _ _ w647 _]
                tunnel: w562 -> [_ _ _ _ _ _ _ _ _ _ _ _ _ w654]
                tunnel: [w579 w585 w591 w595 w600 w605 w612 w619 w625 w632 w635 w643 w648 w652] -> w559
                tunnel: [w580 w584 w589 w596 w601 w606 w613 w620 w626 w631 w637 w642 w647 w653] -> w558
                frame "Carrier BW" {
                  n128 = call "Set_4G_Carrier_Bandwidth.vi"("error in (no error)"=w583, "value"=w580, "Base Station"=w582) -> ("error out"=w581:errorcluster, "Output String"=w579:string)  [unwired: 7 in]
                }
                frame "IMS Enable" {
                  n129 = call "Set_4G_IMS_Enabled.vi"("error in (no error)"=w588, "value"=w584, "Base Station"=w587) -> ("error out"=w586:errorcluster, "Output String"=w585:string)  [unwired: 7 in]
                }
                frame "DL Frequency" {
                  n130 = call "Set_4G_DL_Frequency.vi"("error in (no error)"=w594, "value"=w590, "Base Station"=w593) -> ("error out"=w592:errorcluster, "Output String"=w591:string)  [unwired: 7 in]
                  n131 = call "Number to String.vi"("DecimaL NU\nmber"=w590) -> ("Decimal String"=w589:string)  [unwired: 10 in]
                }
                frame "Duplex Mode" {
                  n132 = call "Set_4G_Duplex_Mode.vi"("error in (no error)"=w599, "value"=w596, "Base Station"=w598) -> ("error out"=w597:errorcluster, "Output String"=w595:string)  [unwired: 7 in]
                }
                frame "Eutra operating band" {
                  n133 = call "Set_4G_EUTRA_Operating_Band.vi"("error in (no error)"=w604, "value"=w601, "Base Station"=w603) -> ("error out"=w602:errorcluster, "Output String"=w600:string)  [unwired: 7 in]
                }
                frame "Measurement report" {
                  n134 = call "String to Number.vi"("Decimal String"=w608) -> ("Decimal Number"=w607:i32)  [unwired: 10 in]
                  n135 = call "Set_4G_Measurement_Report.vi"("error in (no error)"=w611, "value"=w607, "Base Station"=w610) -> ("error out"=w609:errorcluster, "Output String"=w605:string)  [unwired: 7 in]
                  n136 = call "Number to String.vi"("DecimaL NU\nmber"=w607) -> ("Decimal String"=w606:string)  [unwired: 10 in]
                }
                frame "MNC length" {
                  n137 = call "String to Number.vi"("Decimal String"=w615) -> ("Decimal Number"=w614:i32)  [unwired: 10 in]
                  n138 = call "Set_4G_MNC_length.vi"("error in (no error)"=w618, "value"=w614, "Base Station"=w617) -> ("error out"=w616:errorcluster, "Output String"=w612:string)  [unwired: 7 in]
                  n139 = call "Number to String.vi"("DecimaL NU\nmber"=w614) -> ("Decimal String"=w613:string)  [unwired: 10 in]
                }
                frame "MCC" {
                  n140 = call "Number to String.vi"("DecimaL NU\nmber"=w621) -> ("Decimal String"=w620:string)  [unwired: 10 in]
                  n141 = call "Set_4G_Mobile_Country_Code.vi"("error in (no error)"=w624, "value"=w620, "Base Station"=w623) -> ("error out"=w622:errorcluster, "Output String"=w619:string)  [unwired: 7 in]
                }
                frame "MNC" {
                  n142 = call "Number to String.vi"("DecimaL NU\nmber"=w627) -> ("Decimal String"=w626:string)  [unwired: 10 in]
                  n143 = call "Set_4G_Mobile_Network_Code.vi"("error in (no error)"=w630, "value"=w626, "Base Station"=w629) -> ("error out"=w628:errorcluster, "Output String"=w625:string)  [unwired: 7 in]
                }
                frame "network name" {
                  n144 = call "Set_4G_Network_Name.vi"("error in (no error)"=w634, "value"=w631) -> ("error out"=w633:errorcluster, "Output String"=w632:string)  [unwired: 8 in]
                }
                frame "Physical Cell ID" {
                  n145 = call "Set_4G_Physical_Cell_ID.vi"("error in (no error)"=w640, "value"=w636, "Base Station"=w639) -> ("error out"=w638:errorcluster, "Output String"=w635:string)  [unwired: 7 in]
                  n146 = call "Number to String.vi"("DecimaL NU\nmber"=w636) -> ("Decimal String"=w637:string)  [unwired: 10 in]
                }
                frame "Tracking area code" {
                  n147 = call "Set_4G_Tracking_Area_Code.vi"("error in (no error)"=w646, "value"=w641, "Base Station"=w645) -> ("error out"=w644:errorcluster, "Output String"=w643:string)  [unwired: 7 in]
                  n148 = call "Number to String.vi"("DecimaL NU\nmber"=w641) -> ("Decimal String"=w642:string)  [unwired: 10 in]
                }
                frame "Transmission Mode" {
                  n149 = call "Set_4G_Transmission_Mode.vi"("error in (no error)"=w651, "value"=w647, "Base Station"=w650) -> ("error out"=w649:errorcluster, "Output String"=w648:string)  [unwired: 7 in]
                }
                frame "UL frequency" {
                  n150 = call "Set_4G_UL_Frequency.vi"("error in (no error)"=w657, "value"=w654, "Base Station"=w656) -> ("error out"=w655:errorcluster, "Output String"=w652:string)  [unwired: 7 in]
                  n151 = call "Number to String.vi"("DecimaL NU\nmber"=w654) -> ("Decimal String"=w653:string)  [unwired: 10 in]
                }
              }
              n152 = call "Status Update.vi"("Base Station"=w557, "Status Reference"=w560, "Band"="4G", "Status"=w559, "Value"=w558, "error in (no error)"=w578) -> ("value out"=w561:errorcluster)  [unwired: 9 in]
            }
          }
          frame "PHY" {
            w659 = T21 [enum."BCCH modi Coeff", enum."pbch Repetition", enum."pcch Narrowband", enum."pcch pg cycle", enum."pdsch power boost", enum."pdsch Ref power", enum."phich duration", enum."phish resource", enum."prach config index", enum."prach contention resolution", enum."prach initial received target", enum."prach maximum transmission", enum."prach ramping step size", enum."prach response window", enum."prach root sequence", enum."pussh an occassions", enum."pucch cqi num of RB", enum."pucch cs antenna", enum."pucch delta shift", enum."pucch harq max", enum."pucch power offset", enum."pusch alpha", enum."pusch dmrs enable", enum."pusch power offset", enum."srs enable"] items=["BCCH modi Coeff", "pbch Repetition", "pcch Narrowband", "pcch pg cycle", "pdsch power boost", "pdsch Ref power", "phich duration", "phish resource", "prach config index", "prach contention resolution", "prach initial received target", "prach maximum transmission", "prach ramping step size", "prach response window", "prach root sequence", "pussh an occassions", "pucch cqi num of RB", "pucch cs antenna", "pucch delta shift", "pucch harq max", "pucch power offset", "pusch alpha", "pusch dmrs enable", "pusch power offset", "srs enable"] ("Phy 4G")
            n153 = property class="Clust (strict)"(reference=w690, error in=w689) -> (error out=w661:errorcluster, "Value"=w687:T22)  [unwired: 1 out]
            n154 = Unbundle By Name(w687) -> ("PBCH Repetition"=w674:string, "PUCCH Delta Shift"=w673:string, "PUCCH CQI Number of RB"=w675:string, "PHICH Resource"=w676:string, "SRS Enable"=w683:string, "PCCH Paging Cycle"=w679:string, "BCCH Modification Coefficient"=w678:string, "PUSCH Alpha"=w672:string, "PUSCH DMRS Enable"=w670:string, "PHICH Duration"=w684:string, "PUCCH HARQ Max Transmission"=w686:i64, "PCCH Narrowband Count"=w671:string, "PUSCH Power Offset"=w682:i64, "PUCCH Power Offset"=w677:i64, "PDSCH Power Boost"=w680:string, "PUCCH An Occassions"=w681:string, "PUUCH CS Antenna Ports"=w685:string, "PRACH Response Window Size"=w669:string, "PRACH Contention Resolution Timer"=w668:string, "PRACH Ramping Step Size"=w667:string, "PDSCH Reference Power"=w666:i64, "PRACH Root Sequence Index"=w665:i64, "PRACH Maximum Transmissions"=w664:string, "PRACH Initial Received Target Power"=w663:string, "PRACH Configuration Index"=w662:i64)
            n155 = for {
              tunnel: w688 -> [w694]
              tunnel: w686 -> [w704]
              tunnel: w685 -> [w706]
              tunnel: w684 -> [w717]
              tunnel: w683 -> [w699]
              tunnel: w682 -> [w700]
              tunnel: w681 -> [w708]
              tunnel: w680 -> [w719]
              tunnel: w679 -> [w720]
              tunnel: w678 -> [w698]
              tunnel: w677 -> [w703]
              tunnel: w676 -> [w716]
              tunnel: w675 -> [w707]
              tunnel: w674 -> [w697]
              tunnel: w673 -> [w705]
              tunnel: w672 -> [w702]
              tunnel: w671 -> [w721]
              tunnel: w670 -> [w701]
              tunnel: w669 -> [w710]
              tunnel: w668 -> [w714]
              tunnel: w667 -> [w711]
              tunnel: w666 -> [w718]
              tunnel: w665 -> [w709]
              tunnel: w664 -> [w712]
              tunnel: w663 -> [w713]
              tunnel: w662 -> [w715]
              tunnel: w661 -> [w724]
              tunnel: [w696] -> w660
              tunnel: w659 -> [w722] mode=indexing
              tunnel: w658 -> [w695]
              n156 = case shown="\"pbch Repetition\"" w722 {
                tunnel: w724 -> [w729 w735 w740 w745 w751 w757 w763 w768 w774 w779 w784 w789 w794 w799 w805 w811 w817 w823 w829 w835 w841 w846 w852 w858 w864]
                tunnel: [w728 w734 w739 w744 w750 w756 w762 w767 w773 w778 w783 w788 w792 w798 w804 w810 w816 w822 w828 w834 w840 w845 w851 w857 w863] -> w723
                tunnel: w694 -> [w727 w733 w738 w743 w749 w755 w761 w766 w772 w777 w782 w787 w793 w797 w803 w809 w815 w821 w827 w833 w839 w844 w850 w856 w862]
                tunnel: w721 -> [_ _ w736 _ _ _ _ _ _ _ _ _ _ _ _ _ _ _ _ _ _ _ _ _ _]
                tunnel: w720 -> [_ _ _ w741 _ _ _ _ _ _ _ _ _ _ _ _ _ _ _ _ _ _ _ _ _]
                tunnel: w719 -> [_ _ _ _ w746 _ _ _ _ _ _ _ _ _ _ _ _ _ _ _ _ _ _ _ _]
                tunnel: w718 -> [_ _ _ _ _ w753 _ _ _ _ _ _ _ _ _ _ _ _ _ _ _ _ _ _ _]
                tunnel: w717 -> [_ _ _ _ _ _ w758 _ _ _ _ _ _ _ _ _ _ _ _ _ _ _ _ _ _]
                tunnel: w716 -> [_ _ _ _ _ _ _ w764 _ _ _ _ _ _ _ _ _ _ _ _ _ _ _ _ _]
                tunnel: w715 -> [_ _ _ _ _ _ _ _ w770 _ _ _ _ _ _ _ _ _ _ _ _ _ _ _ _]
                tunnel: w714 -> [_ _ _ _ _ _ _ _ _ w775 _ _ _ _ _ _ _ _ _ _ _ _ _ _ _]
                tunnel: w713 -> [_ _ _ _ _ _ _ _ _ _ w780 _ _ _ _ _ _ _ _ _ _ _ _ _ _]
                tunnel: w712 -> [_ _ _ _ _ _ _ _ _ _ _ w785 _ _ _ _ _ _ _ _ _ _ _ _ _]
                tunnel: w711 -> [_ _ _ _ _ _ _ _ _ _ _ _ w790 _ _ _ _ _ _ _ _ _ _ _ _]
                tunnel: w710 -> [_ _ _ _ _ _ _ _ _ _ _ _ _ w795 _ _ _ _ _ _ _ _ _ _ _]
                tunnel: w709 -> [_ _ _ _ _ _ _ _ _ _ _ _ _ _ w801 _ _ _ _ _ _ _ _ _ _]
                tunnel: w708 -> [_ _ _ _ _ _ _ _ _ _ _ _ _ _ _ w806 _ _ _ _ _ _ _ _ _]
                tunnel: w707 -> [_ _ _ _ _ _ _ _ _ _ _ _ _ _ _ _ w812 _ _ _ _ _ _ _ _]
                tunnel: w706 -> [_ _ _ _ _ _ _ _ _ _ _ _ _ _ _ _ _ w818 _ _ _ _ _ _ _]
                tunnel: w705 -> [_ _ _ _ _ _ _ _ _ _ _ _ _ _ _ _ _ _ w824 _ _ _ _ _ _]
                tunnel: w704 -> [_ _ _ _ _ _ _ _ _ _ _ _ _ _ _ _ _ _ _ w830 _ _ _ _ _]
                tunnel: w703 -> [_ _ _ _ _ _ _ _ _ _ _ _ _ _ _ _ _ _ _ _ w836 _ _ _ _]
                tunnel: w702 -> [_ _ _ _ _ _ _ _ _ _ _ _ _ _ _ _ _ _ _ _ _ w842 _ _ _]
                tunnel: w701 -> [_ _ _ _ _ _ _ _ _ _ _ _ _ _ _ _ _ _ _ _ _ _ w847 _ _]
                tunnel: w700 -> [_ _ _ _ _ _ _ _ _ _ _ _ _ _ _ _ _ _ _ _ _ _ _ w853 _]
                tunnel: w699 -> [_ _ _ _ _ _ _ _ _ _ _ _ _ _ _ _ _ _ _ _ _ _ _ _ w859]
                tunnel: w698 -> [w725 _ _ _ _ _ _ _ _ _ _ _ _ _ _ _ _ _ _ _ _ _ _ _ _]
                tunnel: w697 -> [_ w730 _ _ _ _ _ _ _ _ _ _ _ _ _ _ _ _ _ _ _ _ _ _ _]
                tunnel: [w726 w731 w737 w742 w747 w754 w759 w765 w771 w776 w781 w786 w791 w796 w802 w807 w813 w819 w825 w832 w838 w843 w848 w855 w860] -> w692
                tunnel: [w725 w730 w736 w741 w746 w752 w758 w764 w769 w775 w780 w785 w790 w795 w800 w806 w812 w818 w824 w831 w837 w842 w847 w854 w859] -> w691
                frame "BCCH modi Coeff", Default {
                  n157 = call "Set_4G_BCCH_Modification_Coefficient .vi"("error in (no error)"=w729, "value"=w725, "Base Station"=w727) -> ("error out"=w728:errorcluster, "Output String"=w726:string)  [unwired: 7 in]
                }
                frame "pbch Repetition" {
                  n158 = call "String to Number.vi"("Decimal String"=w730) -> ("Decimal Number"=w732:i32)  [unwired: 10 in]
                  n159 = call "Set_4G_PBCH_Repetition.vi"("error in (no error)"=w735, "value"=w732, "Base Station"=w733) -> ("error out"=w734:errorcluster, "Output String"=w731:string)  [unwired: 7 in]
                }
                frame "pcch Narrowband" {
                  n160 = call "Set_4G_PCCH_Narrowband_Count.vi"("error in (no error)"=w740, "value"=w736, "Base Station"=w738) -> ("error out"=w739:errorcluster, "Output String"=w737:string)  [unwired: 7 in]
                }
                frame "pcch pg cycle" {
                  n161 = call "Set_4G_PCCH_Paging_Cycle.vi"("error in (no error)"=w745, "value"=w741, "Base Station"=w743) -> ("error out"=w744:errorcluster, "Output String"=w742:string)  [unwired: 7 in]
                }
                frame "pdsch power boost" {
                  n162 = call "String to Number.vi"("Decimal String"=w746) -> ("Decimal Number"=w748:i32)  [unwired: 10 in]
                  n163 = call "Set_4G_PDSCH_Power_Boost.vi"("error in (no error)"=w751, "value"=w748, "Base Station"=w749) -> ("error out"=w750:errorcluster, "Output String"=w747:string)  [unwired: 7 in]
                }
                frame "pdsch Ref power" {
                  n164 = call "Number to String.vi"("DecimaL NU\nmber"=w753) -> ("Decimal String"=w752:string)  [unwired: 10 in]
                  n165 = call "Set_4G_PDSCH_Reference_Power.vi"("error in (no error)"=w757, "value"=w753, "Base Station"=w755) -> ("error out"=w756:errorcluster, "Output String"=w754:string)  [unwired: 7 in]
                }
                frame "phich duration" {
                  n166 = call "String to Number.vi"("Decimal String"=w758) -> ("Decimal Number"=w760:i32)  [unwired: 10 in]
                  n167 = call "Set_4G_PHICH_Duration.vi"("error in (no error)"=w763, "value"=w760, "Base Station"=w761) -> ("error out"=w762:errorcluster, "Output String"=w759:string)  [unwired: 7 in]
                }
                frame "phish resource" {
                  n168 = call "Set_4G_PHICH_Resource.vi"("error in (no error)"=w768, "value"=w764, "Base Station"=w766) -> ("error out"=w767:errorcluster, "Output String"=w765:string)  [unwired: 7 in]
                }
                frame "prach config index" {
                  n169 = call "Set_4G_PRACH_Configuration_Index.vi"("error in (no error)"=w774, "value"=w770, "Base Station"=w772) -> ("error out"=w773:errorcluster, "Output String"=w771:string)  [unwired: 7 in]
                  n170 = call "Number to String.vi"("DecimaL NU\nmber"=w770) -> ("Decimal String"=w769:string)  [unwired: 10 in]
                }
                frame "prach contention resolution" {
                  n171 = call "Set_4G_PRACH_Contention_Resolution_Timer.vi"("error in (no error)"=w779, "value"=w775, "Base Station"=w777) -> ("error out"=w778:errorcluster, "Output String"=w776:string)  [unwired: 7 in]
                }
                frame "prach initial received target" {
                  n172 = call "Set_4G_PRACH_Initial_Received_Target_Power.vi"("error in (no error)"=w784, "value"=w780, "Base Station"=w782) -> ("error out"=w783:errorcluster, "Output String"=w781:string)  [unwired: 7 in]
                }
                frame "prach maximum transmission" {
                  n173 = call "Set_4G_PRACH_Maximum_Transmissions.vi"("error in (no error)"=w789, "value"=w785, "Base Station"=w787) -> ("error out"=w788:errorcluster, "Output String"=w786:string)  [unwired: 7 in]
                }
                frame "prach ramping step size" {
                  n174 = call "Set_4G_PRACH_Ramping_Step_Size.vi"("error in (no error)"=w794, "value"=w790, "Base Station"=w793) -> ("error out"=w792:errorcluster, "Output String"=w791:string)  [unwired: 7 in]
                }
                frame "prach response window" {
                  n175 = call "Set_4G_PRACH_Response_Window_Size.vi"("error in (no error)"=w799, "value"=w795, "Base Station"=w797) -> ("error out"=w798:errorcluster, "Output String"=w796:string)  [unwired: 7 in]
                }
                frame "prach root sequence" {
                  n176 = call "Set_4G_PRACH_Root_Sequence_Index.vi"("error in (no error)"=w805, "value"=w801, "Base Station"=w803) -> ("error out"=w804:errorcluster, "Output String"=w802:string)  [unwired: 7 in]
                  n177 = call "Number to String.vi"("DecimaL NU\nmber"=w801) -> ("Decimal String"=w800:string)  [unwired: 10 in]
                }
                frame "pussh an occassions" {
                  n178 = call "String to Number.vi"("Decimal String"=w806) -> ("Decimal Number"=w808:i32)  [unwired: 10 in]
                  n179 = call "Set_4G_PUCCH_An_Occassions.vi"("error in (no error)"=w811, "value"=w808, "Base Station"=w809) -> ("error out"=w810:errorcluster, "Output String"=w807:string)  [unwired: 7 in]
                }
                frame "pucch cqi num of RB" {
                  n180 = call "String to Number.vi"("Decimal String"=w812) -> ("Decimal Number"=w814:i32)  [unwired: 10 in]
                  n181 = call "Set_4G_PUCCH_CQI_Number_of_RB.vi"("error in (no error)"=w817, "value"=w814, "Base Station"=w815) -> ("error out"=w816:errorcluster, "Output String"=w813:string)  [unwired: 7 in]
                }
                frame "pucch cs antenna" {
                  n182 = call "String to Number.vi"("Decimal String"=w818) -> ("Decimal Number"=w820:i32)  [unwired: 10 in]
                  n183 = call "Set_4G_PUCCH_CS_Antenna_Ports .vi"("error in (no error)"=w823, "value"=w820, "Base Station"=w821) -> ("error out"=w822:errorcluster, "Output String"=w819:string)  [unwired: 7 in]
                }
                frame "pucch delta shift" {
                  n184 = call "String to Number.vi"("Decimal String"=w824) -> ("Decimal Number"=w826:i32)  [unwired: 10 in]
                  n185 = call "Set_4G_PUCCH_Delta_Shift.vi"("error in (no error)"=w829, "value"=w826, "Base Station"=w827) -> ("error out"=w828:errorcluster, "Output String"=w825:string)  [unwired: 7 in]
                }
                frame "pucch harq max" {
                  n186 = call "Number to String.vi"("DecimaL NU\nmber"=w830) -> ("Decimal String"=w831:string)  [unwired: 10 in]
                  n187 = call "Set_4G_PUCCH_HARQ_Maximum_Transmissions.vi"("error in (no error)"=w835, "value"=w830, "Base Station"=w833) -> ("error out"=w834:errorcluster, "Output String"=w832:string)  [unwired: 7 in]
                }
                frame "pucch power offset" {
                  n188 = call "Set_4G_PUCCH_Power_Offset.vi"("error in (no error)"=w841, "value"=w836, "Base Station"=w839) -> ("error out"=w840:errorcluster, "Output String"=w838:string)  [unwired: 7 in]
                  n189 = call "Number to String.vi"("DecimaL NU\nmber"=w836) -> ("Decimal String"=w837:string)  [unwired: 10 in]
                }
                frame "pusch alpha" {
                  n190 = call "Set_4G_PUSCH_Alpha.vi"("error in (no error)"=w846, "value"=w842, "Base Station"=w844) -> ("error out"=w845:errorcluster, "Output String"=w843:string)  [unwired: 7 in]
                }
                frame "pusch dmrs enable" {
                  n191 = call "String to Number.vi"("Decimal String"=w847) -> ("Decimal Number"=w849:i32)  [unwired: 10 in]
                  n192 = call "Set_4G_PUSCH_DMRS_Enable.vi"("error in (no error)"=w852, "value"=w849, "Base Station"=w850) -> ("error out"=w851:errorcluster, "Output String"=w848:string)  [unwired: 7 in]
                }
                frame "pusch power offset" {
                  n193 = call "Number to String.vi"("DecimaL NU\nmber"=w853) -> ("Decimal String"=w854:string)  [unwired: 10 in]
                  n194 = call "Set_4G_PUSCH_Power_Offset.vi"("error in (no error)"=w858, "value"=w853, "Base Station"=w856) -> ("error out"=w857:errorcluster, "Output String"=w855:string)  [unwired: 7 in]
                }
                frame "srs enable" {
                  n195 = call "String to Number.vi"("Decimal String"=w859) -> ("Decimal Number"=w861:i32)  [unwired: 10 in]
                  n196 = call "Set_4G_SRS_Enable.vi"("error in (no error)"=w864, "value"=w861, "Base Station"=w862) -> ("error out"=w863:errorcluster, "Output String"=w860:string)  [unwired: 7 in]
                }
              }
              n197 = call "Status Update.vi"("Base Station"=w694, "Status Reference"=w695, "Band"="4G", "Status"=w692, "Value"=w691, "error in (no error)"=w723) -> ("value out"=w696:errorcluster)  [unwired: 9 in]
            }
          }
          frame "RRC" {
            w866 = T23 [enum."rlc maxi retransmission", enum."rlc timer poll retransmit", enum."rlc timer reordering", enum."rlc timer status prohibit", enum."rlc poll pdu", enum."rlc poll byte"] items=["rlc maxi retransmission", "rlc poll byte", "rlc poll pdu", "rlc timer poll retransmit", "rlc timer reordering", "rlc timer status prohibit"] ("gprs 4G")
            n198 = property class="Clust (strict)"(reference=w878, error in=w877) -> (error out=w875:errorcluster, "Value"=w876:T24)  [unwired: 1 out]
            n199 = Unbundle By Name(w876) -> ("RLC Maximum Retransmision Threshold"=w869:string, "RLC Timer Poll Retransmit"=w871:i32, "RLC Timer Reordering"=w867:i32, "RLC Timer Status Prohibit"=w872:i32, "RLC Poll PDU"=w868:i32, "RLC Poll Byte"=w870:i32)
            n200 = for {
              tunnel: w873 -> [w882]
              tunnel: w872 -> [w885]
              tunnel: w871 -> [w889]
              tunnel: w870 -> [w887]
              tunnel: w869 -> [w890]
              tunnel: w868 -> [w888]
              tunnel: w867 -> [w886]
              tunnel: w875 -> [w892]
              tunnel: [w884] -> w874
              tunnel: w866 -> [w891] mode=indexing
              tunnel: w865 -> [w883]
              n201 = case shown="\"rlc maxi retransmission\", Default" w891 {
                tunnel: w892 -> [w898 w904 w910 w916 w922 w928]
                tunnel: [w897 w903 w909 w915 w921 w927] -> w893
                tunnel: w882 -> [w896 w902 w908 w914 w920 w926]
                tunnel: w890 -> [w895 _ _ _ _ _]
                tunnel: w889 -> [_ _ _ w913 _ _]
                tunnel: w888 -> [_ _ w907 _ _ _]
                tunnel: w887 -> [_ w901 _ _ _ _]
                tunnel: w886 -> [_ _ _ _ w919 _]
                tunnel: w885 -> [_ _ _ _ _ w924]
                tunnel: [w894 w899 w905 w911 w917 w925] -> w880
                tunnel: [w895 w900 w906 w912 w918 w923] -> w879
                frame "rlc maxi retransmission", Default {
                  n202 = call "Set_4G_RLC_Maximum_Retransmission_Threshold.vi"("error in (no error)"=w898, "value"=w895, "Base Station"=w896) -> ("error out"=w897:errorcluster, "Output String"=w894:string)  [unwired: 7 in]
                }
                frame "rlc poll byte" {
                  n203 = call "Number to String.vi"("DecimaL NU\nmber"=w901) -> ("Decimal String"=w900:string)  [unwired: 10 in]
                  n204 = call "Set_4G_RLC_Poll_Byte.vi"("error in (no error)"=w904, "value"=w901, "Base Station"=w902) -> ("error out"=w903:errorcluster, "Output String"=w899:string)  [unwired: 7 in]
                }
                frame "rlc poll pdu" {
                  n205 = call "Number to String.vi"("DecimaL NU\nmber"=w907) -> ("Decimal String"=w906:string)  [unwired: 10 in]
                  n206 = call "Set_4G_RLC_poll_PDU.vi"("error in (no error)"=w910, "value"=w907, "Base Station"=w908) -> ("error out"=w909:errorcluster, "Output String"=w905:string)  [unwired: 7 in]
                }
                frame "rlc timer poll retransmit" {
                  n207 = call "Set_4G_RLC_Timer_Poll_Retransmit.vi"("error in (no error)"=w916, "value"=w913, "Base Station"=w914) -> ("error out"=w915:errorcluster, "Output String"=w911:string)  [unwired: 7 in]
                  n208 = call "Number to String.vi"("DecimaL NU\nmber"=w913) -> ("Decimal String"=w912:string)  [unwired: 10 in]
                }
                frame "rlc timer reordering" {
                  n209 = call "Set_4G_RLC_Timer_Reordering.vi"("error in (no error)"=w922, "value"=w919, "Base Station"=w920) -> ("error out"=w921:errorcluster, "Output String"=w917:string)  [unwired: 7 in]
                  n210 = call "Number to String.vi"("DecimaL NU\nmber"=w919) -> ("Decimal String"=w918:string)  [unwired: 10 in]
                }
                frame "rlc timer status prohibit" {
                  n211 = call "Set_4G_RLC_Timer_Status_Prohibit.vi"("error in (no error)"=w928, "value"=w924, "Base Station"=w926) -> ("error out"=w927:errorcluster, "Output String"=w925:string)  [unwired: 7 in]
                  n212 = call "Number to String.vi"("DecimaL NU\nmber"=w924) -> ("Decimal String"=w923:string)  [unwired: 10 in]
                }
              }
              n213 = call "Number to String.vi"() -> ()  [unwired: 11 in, 1 out]
              n214 = call "Status Update.vi"("Base Station"=w882, "Status Reference"=w883, "Band"="4G", "Status"=w880, "Value"=w879, "error in (no error)"=w893) -> ("value out"=w884:errorcluster)  [unwired: 9 in]
            }
          }
        }
      }
      frame "gNodeB" {
        n215 = Unbundle By Name(w935) -> ("Ref_Cluster.Status"=w933:refnum<vi>, "Ref_Cluster.NR-PHY"=w936:refnum<vi>, "Ref_Cluster.NR-CELL"=w937:refnum<vi>, "Ref_Cluster.NR-RRC"=w938:refnum<vi>, "Ref_Cluster.NR-SDR"=w939:refnum<vi>, "Ref_Cluster.gNodeB-Data"=w932:refnum<vi>)
        n216 = property class="TabCtl (strict)"(reference=w932, error in=w930) -> (error out=w929:errorcluster, "Value"=w931:enum32{"SDR", "CELL", "PHY", "RRC"})  [unwired: 1 out]
        n217 = case shown="\"RRC\"" w931 {
          tunnel: w929 -> [w941 w955 w1031 w1153 w1289]
          tunnel: [w941 w943 w1015 w1132 w1286] -> w940
          tunnel: w939 -> [_ w956 _ _ _]
          tunnel: w938 -> [_ _ _ _ w1290]
          tunnel: w937 -> [_ _ w1032 _ _]
          tunnel: w936 -> [_ _ _ w1154 _]
          tunnel: w935 -> [_ _ _ _ _]
          tunnel: w934 -> [_ w950 w1028 w1152 w1285]
          tunnel: w933 -> [_ w942 w1012 w1130 w1279]
          frame Default {
          }
          frame "SDR" {
            w951 = T17 [enum."Radio Device", enum."Serial name", enum."dl power", enum."ul ref power", enum."Ul Antennas", enum."Dl Antennas"] items=["Radio Device", "Serial name", "dl power", "ul ref power", "Ul Antennas", "Dl Antennas"] ("Hardware input")
            n218 = property class="Clust (strict)"(reference=w956, error in=w955) -> (error out=w952:errorcluster, "Value"=w954:T25)  [unwired: 1 out]
            n219 = Unbundle By Name(w954) -> ("UL Antennas"=w944:string, "DL Antennas"=w945:string, "Radio Device"=w949:string, "Serail Name"=w948:string, "DL Reference Power"=w953:i32, "UL Reference Power"=w947:i32)
            n220 = for {
              tunnel: w952 -> [w971]
              tunnel: w951 -> [w970] mode=indexing
              tunnel: w950 -> [w960]
              tunnel: T8 "5G" ("Cellular Technology") -> [w959]
              tunnel: w949 -> [w969]
              tunnel: w948 -> [w968]
              tunnel: w953 -> [w966]
              tunnel: w947 -> [w967]
              tunnel: w945 -> [w965]
              tunnel: w944 -> [w964]
              tunnel: [w963] -> w943
              tunnel: w942 -> [w961]
              n221 = case shown="\"ul ref power\"" w970 {
                tunnel: w971 -> [w977 w983 w990 w995 w1002 w1009]
                tunnel: [w976 w982 w989 w994 w1001 w1008] -> w962
                tunnel: w960 -> [w975 w981 w988 w996 w1003 w1010]
                tunnel: w959 -> [w974 w980 w987 w997 w1004 w1011]
                tunnel: w969 -> [w972 _ _ _ _ _]
                tunnel: w968 -> [_ w978 _ _ _ _]
                tunnel: w967 -> [_ _ w985 _ _ _]
                tunnel: w966 -> [_ _ _ w992 _ _]
                tunnel: w965 -> [_ _ _ _ _ w1005]
                tunnel: w964 -> [_ _ _ _ w998 _]
                tunnel: [w973 w979 w986 w993 w999 w1006] -> w958
                tunnel: [w972 w978 w984 w991 w998 w1005] -> w957
                frame "Radio Device", Default {
                  n222 = call "Set_Radio_Device_Name.vi"("error in (no error)"=w977, "value"=w972, "Cellular Technology"=w974, "Base Station"=w975) -> ("error out"=w976:errorcluster, "Output String"=w973:string)  [unwired: 6 in]
                }
                frame "Serial name" {
                  n223 = call "Set_Radio_Device_Serial_Name.vi"("error in (no error)"=w983, "Serial Name"=w978, "Cellular Technology"=w980, "Base Station"=w981) -> ("error out"=w982:errorcluster, "Output String"=w979:string)  [unwired: 6 in]
                }
                frame "dl power" {
                  n224 = call "Number to String.vi"("DecimaL NU\nmber"=w985) -> ("Decimal String"=w984:string)  [unwired: 10 in]
                  n225 = call "Set_Maximum_DL_power.vi"("error in (no error)"=w990, "No of DL antennas Value"=w985, "Cellular Technology"=w987, "Base Station"=w988) -> ("error out"=w989:errorcluster, "Output String"=w986:string)  [unwired: 6 in]
                }
                frame "ul ref power" {
                  n226 = call "Set_Maximum_UL_Reference_power.vi"("error in (no error)"=w995, "Base Station"=w996, "Cellular Technology"=w997, "No of DL antennas Value"=w992) -> ("error out"=w994:errorcluster, "Output String"=w993:string)  [unwired: 6 in]
                  n227 = call "Number to String.vi"("DecimaL NU\nmber"=w992) -> ("Decimal String"=w991:string)  [unwired: 10 in]
                }
                frame "Ul Antennas" {
                  n228 = call "String to Number.vi"("Decimal String"=w998) -> ("Decimal Number"=w1000:i32)  [unwired: 10 in]
                  n229 = call "Set_Number_of_UL_Antennas.vi"("error in (no error)"=w1002, "No of UL antennas Value"=w1000, "Cellular Technology"=w1004, "Base Station"=w1003) -> ("error out"=w1001:errorcluster, "Output String"=w999:string)  [unwired: 6 in]
                }
                frame "Dl Antennas" {
                  n230 = call "String to Number.vi"("Decimal String"=w1005) -> ("Decimal Number"=w1007:i32)  [unwired: 10 in]
                  n231 = call "Set_Number_of_DL_Antennas.vi"("error in (no error)"=w1009, "No of DL antennas Value"=w1007, "Cellular Technology"=w1011, "Base Station"=w1010) -> ("error out"=w1008:errorcluster, "Output String"=w1006:string)  [unwired: 6 in]
                }
              }
              n232 = call "Status Update.vi"("Base Station"=w960, "Status Reference"=w961, "Band"=w959, "Status"=w958, "Value"=w957, "error in (no error)"=w962) -> ("value out"=w963:errorcluster)  [unwired: 9 in]
            }
          }
          frame "CELL" {
            w1013 = T26 [enum."Transmission Mode", enum."Operating Band", enum."Mobile Network Code", enum."Physical Cell ID", enum."SRS", enum."DL offset to Carrier", enum."Tracking Area code", enum."UL Offset to arrier", enum."Carrier Bandwidth", enum."UL Offset to arrier", enum."CSI RS", enum."Subcarrier Spacing", enum."Measurement Report"] items=["Carrier Bandwidth", "CSI RS", "DL offset to Carrier", "Measurement Report", "Mobile Country code", "Mobile Network Code", "Operating Band", "Physical Cell ID", "SRS", "Subcarrier Spacing", "Tracking Area code", "Transmission Mode", "UL Offset to arrier"] ("cell 4G")
            n233 = property class="Clust (strict)"(reference=w1032, error in=w1031) -> (error out=w1029:errorcluster, "Value"=w1030:T27)  [unwired: 1 out]
            n234 = Unbundle By Name(w1030) -> ("Tracking Area Code"=w1027:i64, "Mobile Country Code"=w1025:i64, "Mobile Network Code"=w1023:i64, "Operating Bands"=w1024:string, "Physical Cell ID"=w1022:i64, "DL Offset to Carrier"=w1021:i32, "Subcarrier Spacing"=w1020:string, "UL Offset to Carrier 2"=w1019:i32, "Transmission Mode"=w1018:string, "CSI-RS"=w1026:string, "SRS"=w1017:string, "Measurement Report"=w1016:string, "Carrier Bandwidth"=w1014:string)
            n235 = for {
              tunnel: w1028 -> [w1036]
              tunnel: w1027 -> [w1041]
              tunnel: w1026 -> [w1050]
              tunnel: w1025 -> [w1047]
              tunnel: w1024 -> [w1045]
              tunnel: w1023 -> [w1046]
              tunnel: w1022 -> [w1044]
              tunnel: w1021 -> [w1049]
              tunnel: w1020 -> [w1042]
              tunnel: w1019 -> [w1039]
              tunnel: w1018 -> [w1040]
              tunnel: w1017 -> [w1043]
              tunnel: w1016 -> [w1048]
              tunnel: w1029 -> [w1054]
              tunnel: [w1038] -> w1015
              tunnel: w1013 -> [w1052] mode=indexing
              tunnel: w1014 -> [w1051]
              tunnel: w1012 -> [w1037]
              n236 = case shown="\"Subcarrier Spacing\"" w1052 {
                tunnel: w1054 -> [w1059 w1065 w1071 w1077 w1083 w1089 w1094 w1100 w1106 w1112 w1118 w1123 w1129]
                tunnel: w1036 -> [w1058 w1064 w1070 w1076 w1082 w1088 w1093 w1099 w1105 w1111 w1117 w1122 w1128]
                tunnel: [w1057 w1063 w1069 w1075 w1081 w1087 w1092 w1098 w1104 w1110 w1116 w1121 w1127] -> w1053
                tunnel: w1051 -> [w1055 _ _ _ _ _ _ _ _ _ _ _ _]
                tunnel: w1050 -> [_ w1060 _ _ _ _ _ _ _ _ _ _ _]
                tunnel: w1049 -> [_ _ w1068 _ _ _ _ _ _ _ _ _ _]
                tunnel: w1048 -> [_ _ _ w1072 _ _ _ _ _ _ _ _ _]
                tunnel: w1047 -> [_ _ _ _ w1078 _ _ _ _ _ _ _ _]
                tunnel: w1046 -> [_ _ _ _ _ w1084 _ _ _ _ _ _ _]
                tunnel: w1045 -> [_ _ _ _ _ _ w1090 _ _ _ _ _ _]
                tunnel: w1044 -> [_ _ _ _ _ _ _ w1096 _ _ _ _ _]
                tunnel: w1043 -> [_ _ _ _ _ _ _ _ w1101 _ _ _ _]
                tunnel: w1042 -> [_ _ _ _ _ _ _ _ _ w1107 _ _ _]
                tunnel: w1041 -> [_ _ _ _ _ _ _ _ _ _ w1114 _ _]
                tunnel: w1040 -> [_ _ _ _ _ _ _ _ _ _ _ w1120 _]
                tunnel: w1039 -> [_ _ _ _ _ _ _ _ _ _ _ _ w1124]
                tunnel: [w1056 w1061 w1066 w1073 w1080 w1086 w1091 w1097 w1102 w1108 w1115 w1119 w1126] -> w1034
                tunnel: [w1055 w1060 w1067 w1072 w1079 w1085 w1090 w1095 w1101 w1107 w1113 w1120 w1125] -> w1033
                frame "Carrier Bandwidth" {
                  n237 = call "Set_5G_Carrier_Bandwidth.vi"("error in (no error)"=w1059, "value"=w1055, "Base Station"=w1058) -> ("error out"=w1057:errorcluster, "Output String"=w1056:string)  [unwired: 7 in]
                }
                frame "CSI RS" {
                  n238 = call "String to Number.vi"("Decimal String"=w1060) -> ("Decimal Number"=w1062:i32)  [unwired: 10 in]
                  n239 = call "Set_5G_CSI-RS.vi"("error in (no error)"=w1065, "value"=w1062, "Base Station"=w1064) -> ("error out"=w1063:errorcluster, "Output String"=w1061:string)  [unwired: 7 in]
                }
                frame "DL offset to Carrier" {
                  n240 = call "Set_5G_DL_Offset_to_Carrier.vi"("error in (no error)"=w1071, "value"=w1068, "Base Station"=w1070) -> ("error out"=w1069:errorcluster, "Output String"=w1066:string)  [unwired: 7 in]
                  n241 = call "Number to String.vi"("DecimaL NU\nmber"=w1068) -> ("Decimal String"=w1067:string)  [unwired: 10 in]
                }
                frame "Measurement Report" {
                  n242 = call "String to Number.vi"("Decimal String"=w1072) -> ("Decimal Number"=w1074:i32)  [unwired: 10 in]
                  n243 = call "Set_5G_Measurement_Report.vi"("error in (no error)"=w1077, "value"=w1074, "Base Station"=w1076) -> ("error out"=w1075:errorcluster, "Output String"=w1073:string)  [unwired: 7 in]
                }
                frame "Mobile Country code" {
                  n244 = call "Set_5G_Mobile_Country_Code.vi"("error in (no error)"=w1083, "value"=w1078, "Base Station"=w1082) -> ("error out"=w1081:errorcluster, "Output String"=w1080:string)  [unwired: 7 in]
                  n245 = call "Number to String.vi"("DecimaL NU\nmber"=w1078) -> ("Decimal String"=w1079:string)  [unwired: 10 in]
                }
                frame "Mobile Network Code" {
                  n246 = call "Set_5G_Mobile_Network_Code.vi"("error in (no error)"=w1089, "value"=w1084, "Base Station"=w1088) -> ("error out"=w1087:errorcluster, "Output String"=w1086:string)  [unwired: 7 in]
                  n247 = call "Number to String.vi"("DecimaL NU\nmber"=w1084) -> ("Decimal String"=w1085:string)  [unwired: 10 in]
                }
                frame "Operating Band" {
                  n248 = call "Set_5G_Operating_Band.vi"("error in (no error)"=w1094, "value"=w1090, "Base Station"=w1093) -> ("error out"=w1092:errorcluster, "Output String"=w1091:string)  [unwired: 7 in]
                }
                frame "Physical Cell ID" {
                  n249 = call "Set_5G_Physical_Cell_ID .vi"("error in (no error)"=w1100, "value"=w1096, "Base Station"=w1099) -> ("error out"=w1098:errorcluster, "Output String"=w1097:string)  [unwired: 7 in]
                  n250 = call "Number to String.vi"("DecimaL NU\nmber"=w1096) -> ("Decimal String"=w1095:string)  [unwired: 10 in]
                }
                frame "SRS" {
                  n251 = call "String to Number.vi"("Decimal String"=w1101) -> ("Decimal Number"=w1103:i32)  [unwired: 10 in]
                  n252 = call "Set_5G_SRS.vi"("error in (no error)"=w1106, "value"=w1103, "Base Station"=w1105) -> ("error out"=w1104:errorcluster, "Output String"=w1102:string)  [unwired: 7 in]
                }
                frame "Subcarrier Spacing" {
                  n253 = call "String to Number.vi"("Decimal String"=w1107) -> ("Decimal Number"=w1109:i32)  [unwired: 10 in]
                  n254 = call "Set_5G_Subcarrier_Spacing.vi"("error in (no error)"=w1112, "value"=w1109, "Base Station"=w1111) -> ("error out"=w1110:errorcluster, "Output String"=w1108:string)  [unwired: 7 in]
                }
                frame "Tracking Area code" {
                  n255 = call "Set_5G_Tracking_Area_Code.vi"("error in (no error)"=w1118, "value"=w1114, "Base Station"=w1117) -> ("error out"=w1116:errorcluster, "Output String"=w1115:string)  [unwired: 7 in]
                  n256 = call "Number to String.vi"("DecimaL NU\nmber"=w1114) -> ("Decimal String"=w1113:string)  [unwired: 10 in]
                }
                frame "Transmission Mode" {
                  n257 = call "Set_5G_Transmission_Mode.vi"("error in (no error)"=w1123, "value"=w1120, "Base Station"=w1122) -> ("error out"=w1121:errorcluster, "Output String"=w1119:string)  [unwired: 7 in]
                }
                frame "UL Offset to arrier" {
                  n258 = call "Set_5G_UL_Offset_to_Carrier.vi"("error in (no error)"=w1129, "value"=w1124, "Base Station"=w1128) -> ("error out"=w1127:errorcluster, "Output String"=w1126:string)  [unwired: 7 in]
                  n259 = call "Number to String.vi"("DecimaL NU\nmber"=w1124) -> ("Decimal String"=w1125:string)  [unwired: 10 in]
                }
              }
              n260 = call "Status Update.vi"("Base Station"=w1036, "Status Reference"=w1037, "Band"="5G", "Status"=w1034, "Value"=w1033, "error in (no error)"=w1053) -> ("value out"=w1038:errorcluster)  [unwired: 9 in]
            }
          }
          frame "PHY" {
            w1131 = T28 [enum."PDSCH Reference Power", enum."SSB RSRP Threshold", enum."PRACH Contention Resolution Timer", enum."Preamble Per SSB", enum."Preamble Per SSB Format", enum."UE Power Level Count", enum."RA Response Window", enum."Power Ramp Step Size", enum."Preamble Root Sequence Index", enum."Preamble Transmission  Count", enum."Preamble Received Power", enum."Zero Correlation Zone Configuration", enum."Msg Frequncy Division Multiplexing", enum."PRACH Configuration Index", enum."Preamble Timing Offset", enum."Preamble Format", enum."Resource Restriction Type"] items=["PDSCH Reference Power", "SSB RSRP Threshold", "PRACH Contention Resolution Timer", "Preamble Per SSB", "Preamble Per SSB Format", "UE Power Level Count", "RA Response Window", "Power Ramp Step Size", "Preamble Root Sequence Index", "Preamble Transmission  Count", "Preamble Received Power", "Zero Correlation Zone Configuration", "Msg Frequncy Division Multiplexing", "PRACH Configuration Index", "Preamble Timing Offset", "Preamble Format", "Resource Restriction Type"] ("Phy 5G")
            n261 = property class="Clust (strict)"(reference=w1154, error in=w1153) -> (error out=w1133:errorcluster, "Value"=w1151:T29)  [unwired: 1 out]
            n262 = Unbundle By Name(w1151) -> ("PDSCH Reference Power"=w1138:i64, "SSB RSRP Threshold"=w1137:i64, "PRACH Contention Resolution Timer"=w1139:i64, "Preamble Per SSB"=w1140:i64, "Preamble Per SSB Format"=w1147:i64, "UE Power Level Grant"=w1143:i64, "RA Response Window"=w1142:string, "Power Ramp Step Size"=w1136:string, "Preamble Root Sequence Index"=w1134:string, "Preamble Transmission Count"=w1148:string, "Preamble Received Power"=w1150:i64, "Zero Correlation Zone Configuration"=w1135:i64, "Msg Frequency Division Multiplexing"=w1146:string, "PRACH Configuration Index"=w1141:i64, "Preamble Timing Offset"=w1144:i64, "Preamble Format"=w1145:i64, "Resource Restriction Type"=w1149:string)
            n263 = for {
              tunnel: w1152 -> [w1155]
              tunnel: w1150 -> [w1168]
              tunnel: w1149 -> [w1162]
              tunnel: w1148 -> [w1169]
              tunnel: w1147 -> [w1174]
              tunnel: w1146 -> [w1166]
              tunnel: w1145 -> [w1163]
              tunnel: w1144 -> [w1164]
              tunnel: w1143 -> [w1173]
              tunnel: w1142 -> [w1172]
              tunnel: w1141 -> [w1165]
              tunnel: w1140 -> [w1175]
              tunnel: w1139 -> [w1176]
              tunnel: w1138 -> [w1178]
              tunnel: w1137 -> [w1177]
              tunnel: w1136 -> [w1171]
              tunnel: w1135 -> [w1167]
              tunnel: w1134 -> [w1170]
              tunnel: w1133 -> [w1179]
              tunnel: [w1160] -> w1132
              tunnel: w1131 -> [w1180] mode=indexing
              tunnel: w1130 -> [w1159]
              n264 = case shown="\"Preamble Timing Offset\"" w1180 {
                tunnel: w1179 -> [w1186 w1192 w1198 w1204 w1210 w1216 w1221 w1226 w1231 w1236 w1242 w1248 w1254 w1260 w1266 w1272 w1278]
                tunnel: [w1185 w1191 w1197 w1203 w1209 w1215 w1220 w1225 w1230 w1235 w1241 w1247 w1253 w1259 w1265 w1271 w1277] -> w1161
                tunnel: w1155 -> [w1184 w1190 w1196 w1202 w1208 w1214 w1219 w1224 w1229 w1234 w1240 w1246 w1252 w1258 w1264 w1270 w1276]
                tunnel: w1178 -> [w1181 _ _ _ _ _ _ _ _ _ _ _ _ _ _ _ _]
                tunnel: w1177 -> [_ w1187 _ _ _ _ _ _ _ _ _ _ _ _ _ _ _]
                tunnel: w1176 -> [_ _ w1195 _ _ _ _ _ _ _ _ _ _ _ _ _ _]
                tunnel: w1175 -> [_ _ _ w1199 _ _ _ _ _ _ _ _ _ _ _ _ _]
                tunnel: w1174 -> [_ _ _ _ w1206 _ _ _ _ _ _ _ _ _ _ _ _]
                tunnel: w1173 -> [_ _ _ _ _ w1213 _ _ _ _ _ _ _ _ _ _ _]
                tunnel: w1172 -> [_ _ _ _ _ _ w1217 _ _ _ _ _ _ _ _ _ _]
                tunnel: w1171 -> [_ _ _ _ _ _ _ w1222 _ _ _ _ _ _ _ _ _]
                tunnel: w1170 -> [_ _ _ _ _ _ _ _ w1227 _ _ _ _ _ _ _ _]
                tunnel: w1169 -> [_ _ _ _ _ _ _ _ _ w1232 _ _ _ _ _ _ _]
                tunnel: w1168 -> [_ _ _ _ _ _ _ _ _ _ w1238 _ _ _ _ _ _]
                tunnel: w1167 -> [_ _ _ _ _ _ _ _ _ _ _ w1243 _ _ _ _ _]
                tunnel: w1166 -> [_ _ _ _ _ _ _ _ _ _ _ _ w1249 _ _ _ _]
                tunnel: w1165 -> [_ _ _ _ _ _ _ _ _ _ _ _ _ w1256 _ _ _]
                tunnel: w1164 -> [_ _ _ _ _ _ _ _ _ _ _ _ _ _ w1262 _ _]
                tunnel: w1163 -> [_ _ _ _ _ _ _ _ _ _ _ _ _ _ _ w1268 _]
                tunnel: w1162 -> [_ _ _ _ _ _ _ _ _ _ _ _ _ _ _ _ w1273]
                tunnel: [w1183 w1189 w1194 w1201 w1205 w1211 w1218 w1223 w1228 w1233 w1239 w1245 w1250 w1257 w1261 w1269 w1274] -> w1157
                tunnel: [w1182 w1188 w1193 w1200 w1207 w1212 w1217 w1222 w1227 w1232 w1237 w1244 w1249 w1255 w1263 w1267 w1273] -> w1156
                frame "PDSCH Reference Power", Default {
                  n265 = call "Set_5G_PDSCH_Reference_Power.vi"("error in (no error)"=w1186, "value"=w1181, "Base Station"=w1184) -> ("error out"=w1185:errorcluster, "Output String"=w1183:string)  [unwired: 7 in]
                  n266 = call "Number to String.vi"("DecimaL NU\nmber"=w1181) -> ("Decimal String"=w1182:string)  [unwired: 10 in]
                }
                frame "SSB RSRP Threshold" {
                  n267 = call "Set_5G_SSB_RSRP_Threshold.vi"("error in (no error)"=w1192, "value"=w1187, "Base Station"=w1190) -> ("error out"=w1191:errorcluster, "Output String"=w1189:string)  [unwired: 7 in]
                  n268 = call "Number to String.vi"("DecimaL NU\nmber"=w1187) -> ("Decimal String"=w1188:string)  [unwired: 10 in]
                }
                frame "PRACH Contention Resolution Timer" {
                  n269 = call "Number to String.vi"("DecimaL NU\nmber"=w1195) -> ("Decimal String"=w1193:string)  [unwired: 10 in]
                  n270 = call "Set_5G_PRACH_Contention_Resolution_Timer.vi"("error in (no error)"=w1198, "value"=w1193, "Base Station"=w1196) -> ("error out"=w1197:errorcluster, "Output String"=w1194:string)  [unwired: 7 in]
                }
                frame "Preamble Per SSB" {
                  n271 = call "Set_5G_Preamble_per_SSB.vi"("error in (no error)"=w1204, "value"=w1199, "Base Station"=w1202) -> ("error out"=w1203:errorcluster, "Output String"=w1201:string)  [unwired: 7 in]
                  n272 = call "Number to String.vi"("DecimaL NU\nmber"=w1199) -> ("Decimal String"=w1200:string)  [unwired: 10 in]
                }
                frame "Preamble Per SSB Format" {
                  n273 = call "Set_5G_Preamble_per_SSB_Format.vi"("error in (no error)"=w1210, "value"=w1206, "Base Station"=w1208) -> ("error out"=w1209:errorcluster, "Output String"=w1205:string)  [unwired: 7 in]
                  n274 = call "Number to String.vi"("DecimaL NU\nmber"=w1206) -> ("Decimal String"=w1207:string)  [unwired: 10 in]
                }
                frame "UE Power Level Count" {
                  n275 = call "Set_5G_UE_Power_Level_Grant.vi"("error in (no error)"=w1216, "value"=w1213, "Base Station"=w1214) -> ("error out"=w1215:errorcluster, "Output String"=w1211:string)  [unwired: 7 in]
                  n276 = call "Number to String.vi"("DecimaL NU\nmber"=w1213) -> ("Decimal String"=w1212:string)  [unwired: 10 in]
                }
                frame "RA Response Window" {
                  n277 = call "Set_5G_RA_Response_Window.vi"("error in (no error)"=w1221, "value"=w1217, "Base Station"=w1219) -> ("error out"=w1220:errorcluster, "Output String"=w1218:string)  [unwired: 7 in]
                }
                frame "Power Ramp Step Size" {
                  n278 = call "Set_5G_Power_ramp_Step_Size.vi"("error in (no error)"=w1226, "value"=w1222, "Base Station"=w1224) -> ("error out"=w1225:errorcluster, "Output String"=w1223:string)  [unwired: 7 in]
                }
                frame "Preamble Root Sequence Index" {
                  n279 = call "Set_5G_Preamble_Root_Sequence_Index.vi"("error in (no error)"=w1231, "value"=w1227, "Base Station"=w1229) -> ("error out"=w1230:errorcluster, "Output String"=w1228:string)  [unwired: 7 in]
                }
                frame "Preamble Transmission  Count" {
                  n280 = call "Set 5G Preamble  Transmission Count.vi"("error in (no error)"=w1236, "value"=w1232, "Base Station"=w1234) -> ("error out"=w1235:errorcluster, "Output String"=w1233:string)  [unwired: 7 in]
                }
                frame "Preamble Received Power" {
                  n281 = call "Set 5G Preamble  Received Power.vi"("error in (no error)"=w1242, "value"=w1238, "Base Station"=w1240) -> ("error out"=w1241:errorcluster, "Output String"=w1239:string)  [unwired: 7 in]
                  n282 = call "Number to String.vi"("DecimaL NU\nmber"=w1238) -> ("Decimal String"=w1237:string)  [unwired: 10 in]
                }
                frame "Zero Correlation Zone Configuration" {
                  n283 = call "Set 5G Zero Correlation Zone Configuration.vi"("error in (no error)"=w1248, "value"=w1243, "Base Station"=w1246) -> ("error out"=w1247:errorcluster, "Output String"=w1245:string)  [unwired: 7 in]
                  n284 = call "Number to String.vi"("DecimaL NU\nmber"=w1243) -> ("Decimal String"=w1244:string)  [unwired: 10 in]
                }
                frame "Msg Frequncy Division Multiplexing" {
                  n285 = call "String to Number.vi"("Decimal String"=w1249) -> ("Decimal Number"=w1251:i32)  [unwired: 10 in]
                  n286 = call "Set 5G Msg1 Frequency Division Multiplexing.vi"("error in (no error)"=w1254, "value"=w1251, "Base Station"=w1252) -> ("error out"=w1253:errorcluster, "Output String"=w1250:string)  [unwired: 7 in]
                }
                frame "PRACH Configuration Index" {
                  n287 = call "Set 5G  PRACH Configuration Index.vi"("error in (no error)"=w1260, "value"=w1256, "Base Station"=w1258) -> ("error out"=w1259:errorcluster, "Output String"=w1257:string)  [unwired: 7 in]
                  n288 = call "Number to String.vi"("DecimaL NU\nmber"=w1256) -> ("Decimal String"=w1255:string)  [unwired: 10 in]
                }
                frame "Preamble Timing Offset" {
                  n289 = call "Set 5G  Preamble Timing Offset.vi"("error in (no error)"=w1266, "value"=w1262, "Base Station"=w1264) -> ("error out"=w1265:errorcluster, "Output String"=w1261:string)  [unwired: 7 in]
                  n290 = call "Number to String.vi"("DecimaL NU\nmber"=w1262) -> ("Decimal String"=w1263:string)  [unwired: 10 in]
                }
                frame "Preamble Format" {
                  n291 = call "Set 5G Preamble Format.vi"("error in (no error)"=w1272, "value"=w1268, "Base Station"=w1270) -> ("error out"=w1271:errorcluster, "Output String"=w1269:string)  [unwired: 7 in]
                  n292 = call "Number to String.vi"("DecimaL NU\nmber"=w1268) -> ("Decimal String"=w1267:string)  [unwired: 10 in]
                }
                frame "Resource Restriction Type" {
                  n293 = call "String to Number.vi"("Decimal String"=w1273) -> ("Decimal Number"=w1275:i32)  [unwired: 10 in]
                  n294 = call "Set 5G Resource Restriction Type .vi"("error in (no error)"=w1278, "value"=w1275, "Base Station"=w1276) -> ("error out"=w1277:errorcluster, "Output String"=w1274:string)  [unwired: 7 in]
                }
              }
              n295 = call "Status Update.vi"("Base Station"=w1155, "Status Reference"=w1159, "Band"="5G", "Status"=w1157, "Value"=w1156, "error in (no error)"=w1161) -> ("value out"=w1160:errorcluster)  [unwired: 9 in]
            }
          }
          frame "RRC" {
            w1280 = T30 [enum."Ciphering Algorithms for SRB", enum."Integrity Algorithms for SRB", enum."Ciphering Algorithms for DRB", enum."Integrity Algorithms for DRB"] items=["Ciphering Algorithms for SRB", "Integrity Algorithms for SRB", "Ciphering Algorithms for DRB", "Integrity Algorithms for DRB"] ("gprs 4G")
            n296 = property class="Clust (strict)"(reference=w1290, error in=w1289) -> (error out=w1287:errorcluster, "Value"=w1288:T31)  [unwired: 1 out]
            n297 = Unbundle By Name(w1288) -> ("Ciphering Algorithms for SRB"=w1282:string, "Integrity Algorithms for SRB"=w1283:string, "Ciphering Algorithms for DRB"=w1281:string, "Integrity Algorithms for DRB"=w1284:string)
            n298 = for {
              tunnel: w1285 -> [w1294]
              tunnel: w1284 -> [w1297]
              tunnel: w1283 -> [w1298]
              tunnel: w1282 -> [w1300]
              tunnel: w1281 -> [w1299]
              tunnel: w1287 -> [w1302]
              tunnel: [w1296] -> w1286
              tunnel: w1280 -> [w1301] mode=indexing
              tunnel: w1279 -> [w1295]
              n299 = case shown="\"Integrity Algorithms for DRB\"" w1301 {
                tunnel: w1302 -> [w1308 w1313 w1319 w1325]
                tunnel: [w1307 w1312 w1318 w1324] -> w1303
                tunnel: w1294 -> [w1306 w1311 w1317 w1323]
                tunnel: w1300 -> [w1304 _ _ _]
                tunnel: w1299 -> [_ _ w1315 _]
                tunnel: w1298 -> [_ w1310 _ _]
                tunnel: w1297 -> [_ _ _ w1320]
                tunnel: [w1305 w1309 w1314 w1321] -> w1292
                tunnel: [w1304 w1310 w1315 w1320] -> w1291
                frame "Ciphering Algorithms for SRB", Default {
                  n300 = call "Set_5G_Ciphering_Algorithms_for_SRB.vi"("error in (no error)"=w1308, "value"=w1304, "Base Station"=w1306) -> ("error out"=w1307:errorcluster, "Output String"=w1305:string)  [unwired: 7 in]
                }
                frame "Integrity Algorithms for SRB" {
                  n301 = call "Set_5G_Integrity_Algorithms_for_SRB.vi"("error in (no error)"=w1313, "value"=w1310, "Base Station"=w1311) -> ("error out"=w1312:errorcluster, "Output String"=w1309:string)  [unwired: 7 in]
                }
                frame "Ciphering Algorithms for DRB" {
                  n302 = call "String to Number.vi"("Decimal String"=w1315) -> ("Decimal Number"=w1316:i32)  [unwired: 10 in]
                  n303 = call "Set_5G_Ciphering_Algorithms_for_DRB.vi"("error in (no error)"=w1319, "value"=w1316, "Base Station"=w1317) -> ("error out"=w1318:errorcluster, "Output String"=w1314:string)  [unwired: 7 in]
                }
                frame "Integrity Algorithms for DRB" {
                  n304 = call "String to Number.vi"("Decimal String"=w1320) -> ("Decimal Number"=w1322:i32)  [unwired: 10 in]
                  n305 = call "Set_5G_Integrity_Algorithms_for_DRB.vi"("error in (no error)"=w1325, "value"=w1322, "Base Station"=w1323) -> ("error out"=w1324:errorcluster, "Output String"=w1321:string)  [unwired: 7 in]
                }
              }
              n306 = call "Status Update.vi"("Base Station"=w1294, "Status Reference"=w1295, "Band"="5G", "Status"=w1292, "Value"=w1291, "error in (no error)"=w1303) -> ("value out"=w1296:errorcluster)  [unwired: 9 in]
            }
          }
        }
      }
    }
  }
  "error out" <- w3
